vi "TLB Native Dynamic Events ver 0.16a.vi"() -> ()   [LabVIEW 2018]
uses:
  Labview Training Phase 2/Enum Controls/States for Action Engine.ctl
  TLB Type Definitions/State Type Definitions.ctl
  TLB Type Definitions/Intruction Type Definitions.ctl
  TLB Type Definitions/Encoder cluster.ctl
  TLB Type Definitions/PING CLUSTER.ctl
  <vilib>/Studica/Studica Toolkit/NavX/NavX.lvlib
  <vilib>/Studica/Studica Toolkit/Background/DIO Channel.ctl
  Underlying VI's/NavX VI/navX type def.ctl
  <vilib>/myRIO/Instrument Drivers/Utilities/Utilities.lvlib
  <vilib>/Studica/Studica Toolkit/Background/I2C Channel.ctl
  TLB Type Definitions/Vision cluster.ctl
  <vilib>/NI_Real-Time Target Support.lvlib
  TLB Type Definitions/Stepper cluster.ctl
  Experimental VI's/Archived VI's/MOTOR CONTROL NO PID Type Def.ctl
  Underlying VI's/I2C Master VI/I2C MASTER Type Def.ctl
  Underlying VI's/I2C Master VI/I2C_MASTER_WRITE_NEW Type Def.ctl
  <vilib>/userdefined/High Color/IMAQdx.ctl
  Underlying VI's/I2C Master VI/Arduino_Interfacing.ctl
  TLB Type Definitions/Yaw Cluster.ctl
  TLB Type Definitions/Time cluster.ctl
  TLB Type Definitions/Y Stepper cluster.ctl
  Underlying VI's/Modified webcam FGV/Webcam AE.ctl
  Underlying VI's/Elasped Timer/Elapsed timer control.ctl
  Underlying VI's/Motor Control VI with PID/MOTOR CONTROL WITH PID AE DATA MODE TYPE DEF.ctl
  Underlying VI's/Motor Control VI with PID/MOTOR CONTROL WITH PID AE DIRECTION TYPE DEF.ctl
  TLB Type Definitions/IR Sensor Type Def.ctl
  <vilib>/myRIO/Common/Instrument Driver Framework/myRIO v1.0/AI/typedefs/AI Channels Enum.ctl
  <vilib>/myRIO/Common/Instrument Driver Framework/myRIO v1.0/AI/typedefs/AI Channels List.ctl
  <vilib>/Utility/RT CPU Load.ctl
panel:
  out "Left IR Sensor":dbl
  out "Obstacle detected":bool
  out "Speed & distance":T1
  out "Object Center Coordinates":cluster{"x":sgl, "y":sgl}
  out "Object detection cluster":T2
  out "Time up flag":bool
  out "Task selection":u8
  in  "Object recognition mode":enum16{"Ball", "Soap", "Gel", "Pipe", "None"}(ring)
  out "NavX Readings":T3
  out "Arduino Data":T4
  out "CPU loads":T5[](array[typedef]) {"ISR (%)" format="%#.2f"; "Idle (%)" format="%#.2f"; "Background (%)" format="%#.2f"; "Normal (%)" format="%#.2f"; "Above Normal (%)" format="%#.2f"; "High (%)" format="%#.2g"; "Timed Structures (%)" format="%#.2g"; "Time Critical (%)" format="%#.2g"; "Total (%)" format="%#.2g"}
  out "TASK ENABLE":bool
  out "Rising Edge":bool
  in  "Green LED":bool
  out "I2C Error":errorcluster
  out "State Logic":T6=enum."Startup"
  out "elements":T7[](array[typedef])
  in  "STOP TASK":bool
  in  "OK Button":bool
  in  "STOP":bool
  out "error out":errorcluster
  out "Action Queue Items":i32
  out "State Logic Queue Items":i32
  out "Action Queues items":string[](array[string])=["Hardware reset", "Software reset", ""]
  out "Action State":string
  # "System Health Status Update"
  # "VISION"
  # "TLB FRAMEWORK STATUS"
  # "Test Programme written by Calvin Loke    Dated: 28 Aug 2019\nTest Programme revised by Dr Alex See   Dated 30 Aug 2019\n\nRevision date: 20/03/2020\nProgramme version:   TLB Native Dynamic Events ver 0.14a"
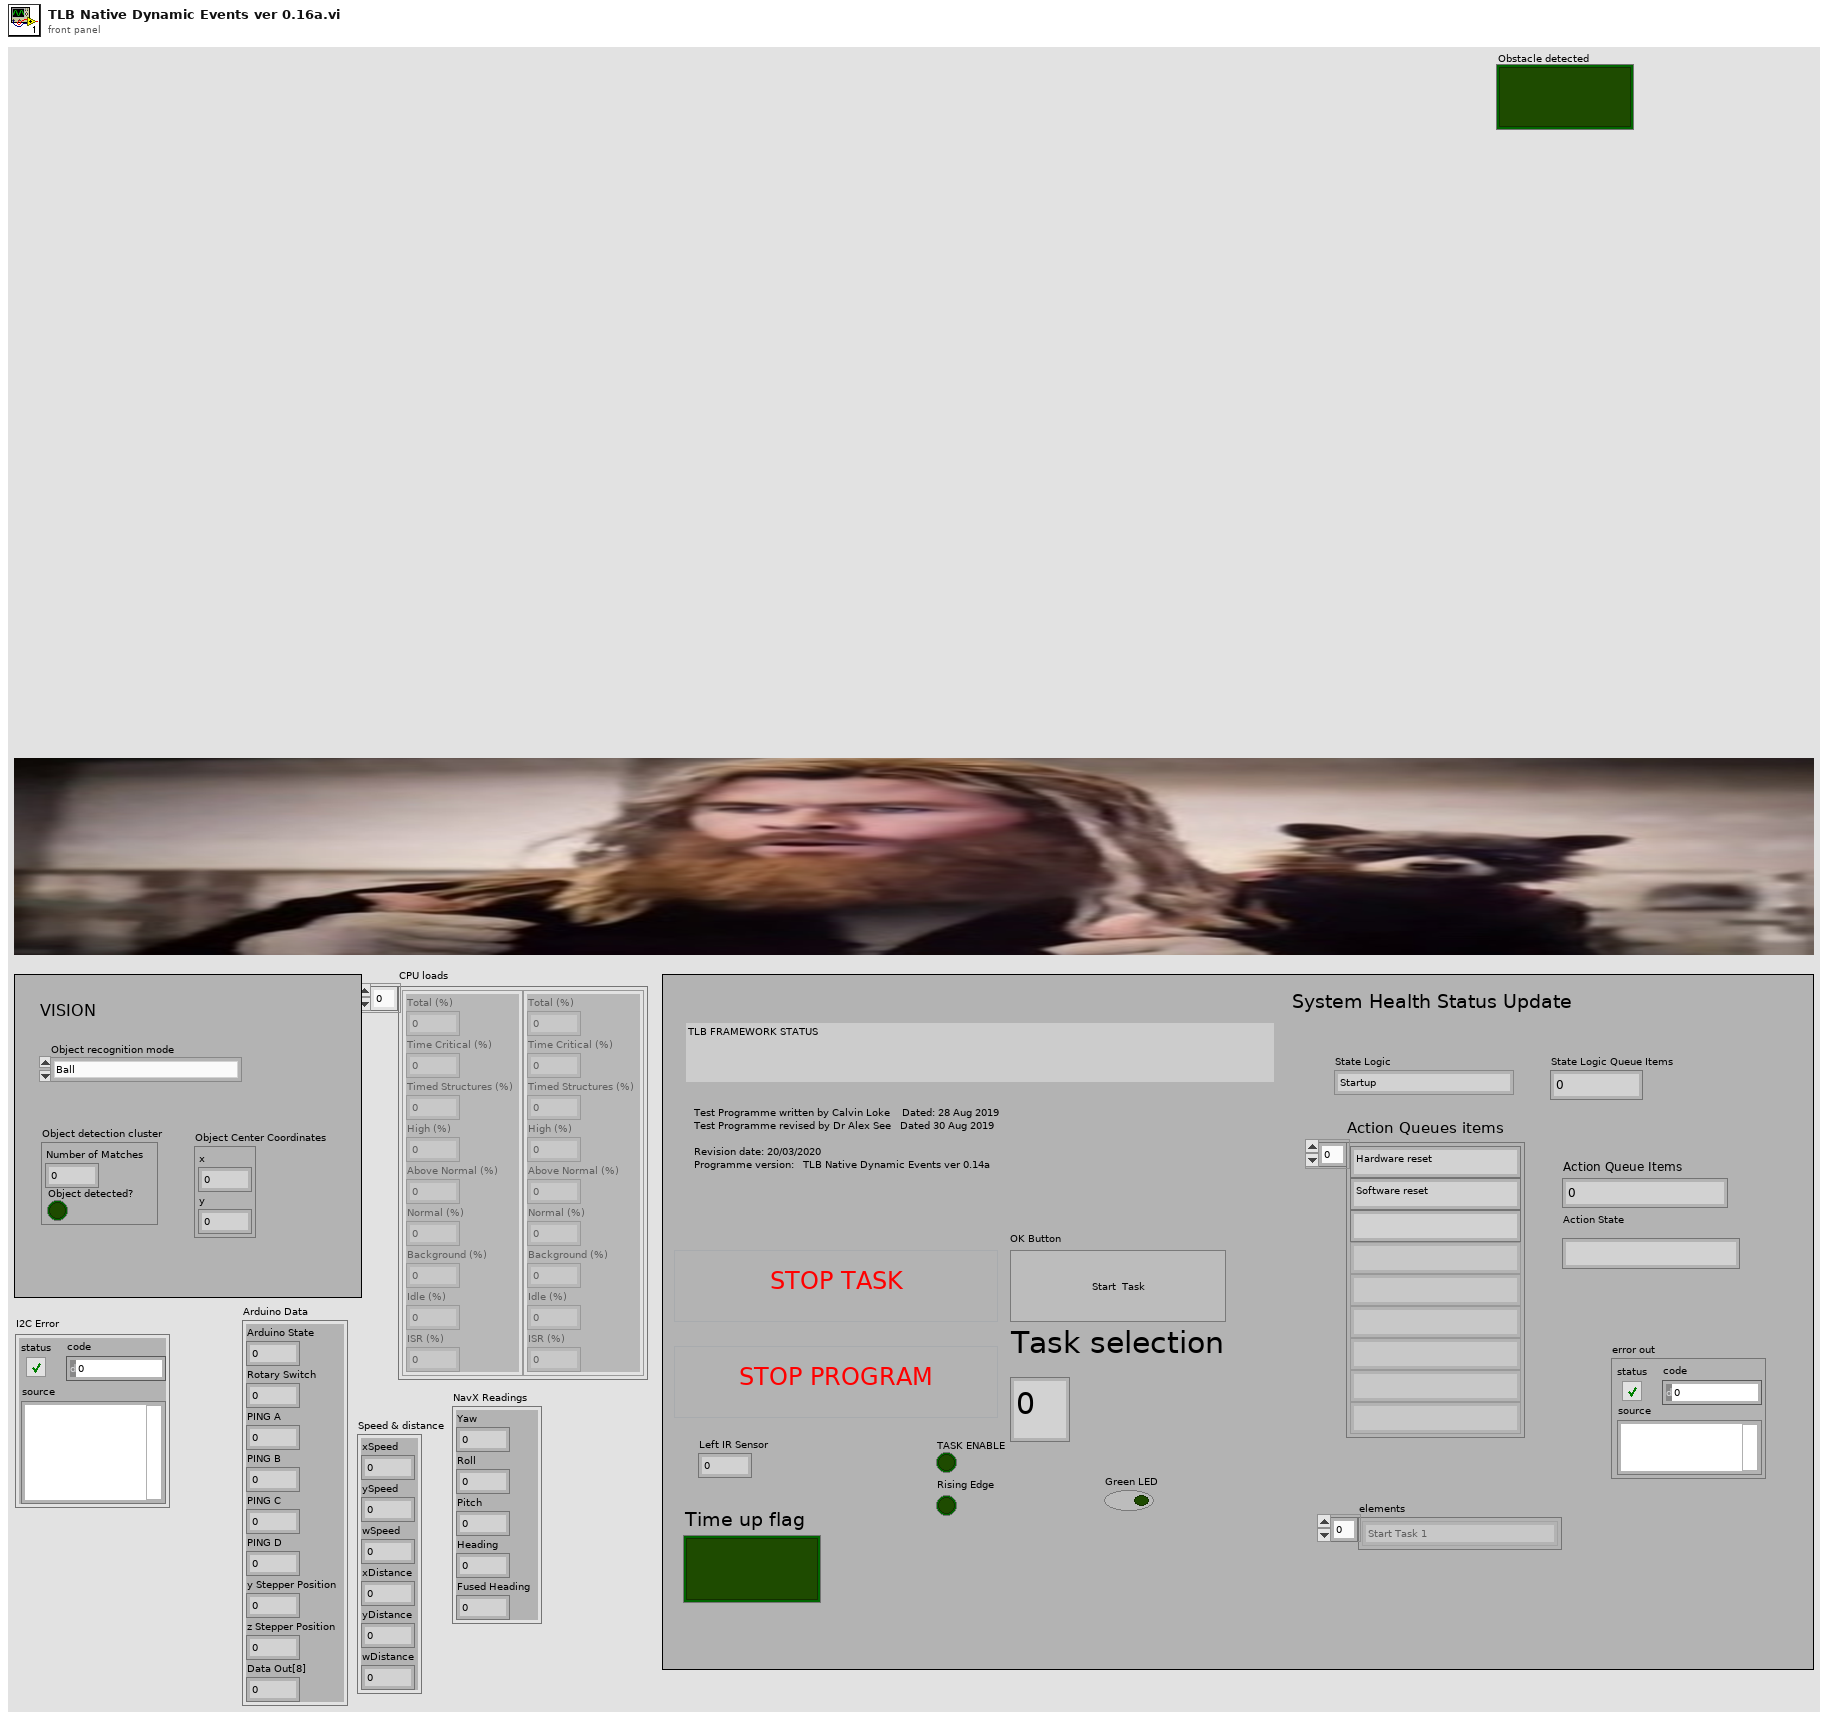
[diagram p1: front panel]
types:
  T1 = cluster{"xSpeed":dbl, "ySpeed":dbl, "wSpeed":dbl, "xDistance":dbl, "yDistance":dbl, "wDistance":dbl}
  T2 = cluster{"Number of Matches":i32, "Object detected?":bool}
  T3 = cluster{"Yaw":dbl, "Roll":dbl, "Pitch":dbl, "Heading":dbl, "Fused Heading":dbl}
  T4 = cluster{"Arduino State":u8, "Rotary Switch":u8, "PING A":u8, "PING B":u8, "PING C":u8, "PING D":u8, "y Stepper Position":u8, "z Stepper Position":u8, "Data Out[8]":u8}
  T5 = typedef "NI_Real-Time Target Support.lvlib/RT CPU Load.ctl" = cluster{"Total (%)":dbl, "Time Critical (%)":dbl, "Timed Structures (%)":dbl, "High (%)":dbl, "Above Normal (%)":dbl, "Normal (%)":dbl, "Background (%)":dbl, "Idle (%)":dbl, "ISR (%)":dbl}
  T6 = typedef "State Type Definitions.ctl" = enum16{"None", "Startup", "Move to Angle", "True Stop", "Idle", "Shutdown", "Task 1A", "Task 1B", "Task 2:Raise Arm", "Task 2:Sensor Mode", "Task 2:Reverse Mode", "Task 3", "Task 4_A", "Task 4_B", "Task 4_C", "Task 4_D", "Task 5A", "Task 5B", "Task 5C", "Task 5D", "Task 5E: POSITION ARM", "Task 5F: ARM GRAB HEIGHT", "Task 5G: CLOSE CLAW", "Task 5H: RAISE ARM", "Task 6_A", "Task 6_B", "Task 7", "Task 8A: RAISE ARM", "Task 8B: MOVE TO BOX", "Task 8C: CAM BURST", "Task 8D: PROCESS IMAGE", "Task 8E: ROBOT ADJUST", "Task 8F: CAM BURST 2", "Task 8G: PROCESS IMAGE 2", "Task 8H: ARM ADJUST", "Task 8I: ARM GRAB HEIGHT", "Task 8J: CLOSE CLAW", "Task 8K: RAISE MY SWORD", "Task 9A: Raise Arm", "Task 9B: Rotate to Angle", "Task 9C: Detect Box", "Task 9D: MOVE FORWARD", "Task 9E: MOVE LEFT", "Task 9F: SCAN IMAGE", "Task 9G: PROCESS COLOUR", "Task 9H: MOVE RIGHT", "Task 9I: SCAN IMAGE", "Task 9J: PROCESS COLOUR", "Task 9K: ROTATE 90 CW", "Task 9L: MOVE FORWARD", "Task 9M: MOVE RIGHT", "Task 9N: SCAN IMAGE", "Task 9O: PROCESS COLOUR", "Task 9P: MOVE RIGHT", "Task 9Q: SCAN IMAGE", "Task 9R: PROCESS COLOUR", "Task A1: Raise Arm", "Task A2: Rotate to Angle", "Task A3: Move Forward", "Task A4: Rotate CW 90"}
  T7 = typedef "Intruction Type Definitions.ctl" = enum16{"None", "Start Task 1", "Start Task 2", "Start Task 3", "Start Task 4", "Start Task 5", "Start Task 6", "Start Task 7", "Start Task 8 - BALL", "Start Task 8 - Gel", "Start Task 8 - Pipe", "Start Task 8 - Soap", "Start Task 9", "Start Task A", "Start Task B", "Exit"}
  T8 = typedef "IR Sensor Type Def.ctl" = cluster{"Left IR Sensor":dbl, "Arm IR Sensor":dbl, "Bottom IR Sensor":dbl}
  T9 = typedef "Y Stepper cluster.ctl" = cluster{"yStepper desired":u8}
  T10 = typedef "Time cluster.ctl" = cluster{"Time up flag":bool, "SET TIME TO CHECK":dbl}
  T11 = typedef "Yaw Cluster.ctl" = cluster{"Yaw":dbl, "Compass":dbl}
  T12 = typedef "Stepper cluster.ctl" = cluster{"y Stepper Position":u8, "z Stepper Position":u8}
  T13 = typedef "DIO Channel.ctl" = enum16{"Not Connected", "A/DIO1", "A/DIO2", "A/DIO3", "A/DIO4", "A/DIO5", "A/DIO6", "A/DIO7", "A/DIO13", "B/DIO1", "B/DIO2", "B/DIO3", "B/DIO4", "B/DIO5", "B/DIO6", "B/DIO7", "B/DIO13", "C/DIO0", "C/DIO1", "C/DIO2", "C/DIO3", "C/DIO4", "C/DIO5", "C/DIO6", "C/DIO7"}
  T14 = typedef "Vision cluster.ctl" = cluster{"Recognized Object":bool, "Object X coordinate":dbl, "Object Y coordinate":dbl}
  T15 = typedef "PING CLUSTER.ctl" = cluster{"PING_A":u8, "PING_B":u8, "PING_C":u8, "PING_D":u8}
  T16 = typedef "Encoder cluster.ctl" = cluster{"xDistance":dbl, "yDistance":dbl, "wDistance":dbl}
  T17 = cluster{"DIO Channel":T13, "FPGA VI Reference Out":refnum<k20>}
  T18 = typedef "navX type def.ctl" = enum16{"Get i2C reference", "Read Values", "Zero Yaw"}
  T19 = typedef "Arduino_Interfacing.ctl" = enum16{"Initialize", "Write to Arduino", "Read From Arduino"}
  T20 = typedef "I2C Channel.ctl" = enum16{"Not Connected", "A", "B"}
  T21 = typedef "States for Action Engine.ctl" = enum16{"Initialize", "Write", "Read"}
  T22 = cluster{"I2C Ref Out":cluster{"I2C Channel":T20, "FPGA VI Reference Out":refnum<k20>}, "Connected":bool, "Slave Address (7-bit)":u8, "Registry":u8[]}
  T23 = typedef "IMAQ Image.ctl" = refnum<image>
  T24 = typedef "State Type Definitions.ctl" = enum16{"None", "Startup", "Move to Angle", "True Stop", "Idle", "Shutdown", "Task 1", "Task 2:Raise Arm", "Task 2:Sensor Mode", "Task 3", "Task 4_A", "Task 4_B", "Task 4_C", "Task 4_D", "Task 5_A", "Task 5 _B", "Task 5_C", "Task 5_D", "Task 5_D_Error", "Task 5D_Error_Right", "Task 5D_Error_Left", "Task 5_E", "Task 5_F", "Task 5F_Error", "Task 5G", "Task 5H", "Task 5I", "Task 6_A", "Task 6_B", "Task 7", "Task 8", "Task 9A: Raise Arm", "Task 9B: Rotate to Angle", "Task 9C: Rotation alignmnet", "Task B"}
  T25 = typedef "MOTOR CONTROL WITH PID AE DIRECTION TYPE DEF.ctl" = enum16{"y-axis movement", "x-axis movement", "rotation", "stop", "reset encoders"}
  T26 = typedef "MOTOR CONTROL WITH PID AE DATA MODE TYPE DEF.ctl" = enum16{"Init AE", "Write to AE", "Read from AE"}
  T27 = typedef "Elapsed timer control.ctl" = enum16{"Start", "Pause", "Initialize"}
  T28 = typedef "I2C_MASTER_WRITE_NEW Type Def.ctl" = enum16{"Ultrasonic sensors", "Stepper origin", "zStepper 13.3k", "zStepper 13k", "zStepper 12k", "zStepper 11k", "zStepper 10k", "zStepper 9k", "zStepper 8k", "zStepper 7k", "zStepper 6k", "zStepper 5k", "zStepper 4k", "zStepper 3k", "zStepper 2k", "zStepper 1k", "zStepper 900", "zStepper 800", "zStepper 700", "zStepper 600", "zStepper 500", "zStepper 400", "zStepper 300", "zStepper 200", "zStepper 100", "zStepper 0", "yStepper control", "Open Claw", "Close Claw", "Soft Reset"}
  T29 = typedef "Webcam AE.ctl" = enum16{"Initialize Camera", "Open Camera", "Continuous Acquisition", "Close Camera", "Retrieve Image", "Dispose Camera Image Buffer"}
  T30 = typedef "IMAQdx.ctl" = refnum<k21>
  T31 = typedef "Webcam AE.ctl" = enum16{"Initialize Camera", "Open Camera", "Continuous Acquisition", "Close Camera", "Retrieve Image", "Dispose Image Buffers"}
  T32 = typedef "MOTOR CONTROL NO PID Type Def.ctl" = enum16{"Init", "Front Back", "Left Right", "Rotate", "Stop", "Latch"}
  T33 = typedef "AI Channels List.ctl" = T34[]
  T34 = typedef "AI Channels Enum.ctl" = enum16{"Not Connected", "AudioIn/Left", "AudioIn/Right", "C/AI0", "C/AI1", "A/AI0", "A/AI1", "A/AI2", "A/AI3", "A/AI4", "A/AI5", "A/AI6", "A/AI7", "B/AI0", "B/AI1", "B/AI2", "B/AI3", "B/AI4", "B/AI5", "B/AI6", "B/AI7", "AI/AI0", "AI/AI1", "AI/AI2", "AI/AI3", "A/AI0 (DIFF)", "A/AI1 (DIFF)", "A/AI2 (DIFF)", "A/AI3 (DIFF)", "B/AI0 (DIFF)", "B/AI1 (DIFF)", "B/AI2 (DIFF)", "B/AI3 (DIFF)"}
  T35 = typedef "I2C MASTER Type Def.ctl" = enum16{"Last State", "Mode 0", "Mode 1", "Mode 2", "Mode 3", "Mode 4", "Mode 5", "Mode 6", "Mode 7", "Mode 8", "Mode 9", "Mode 10"}
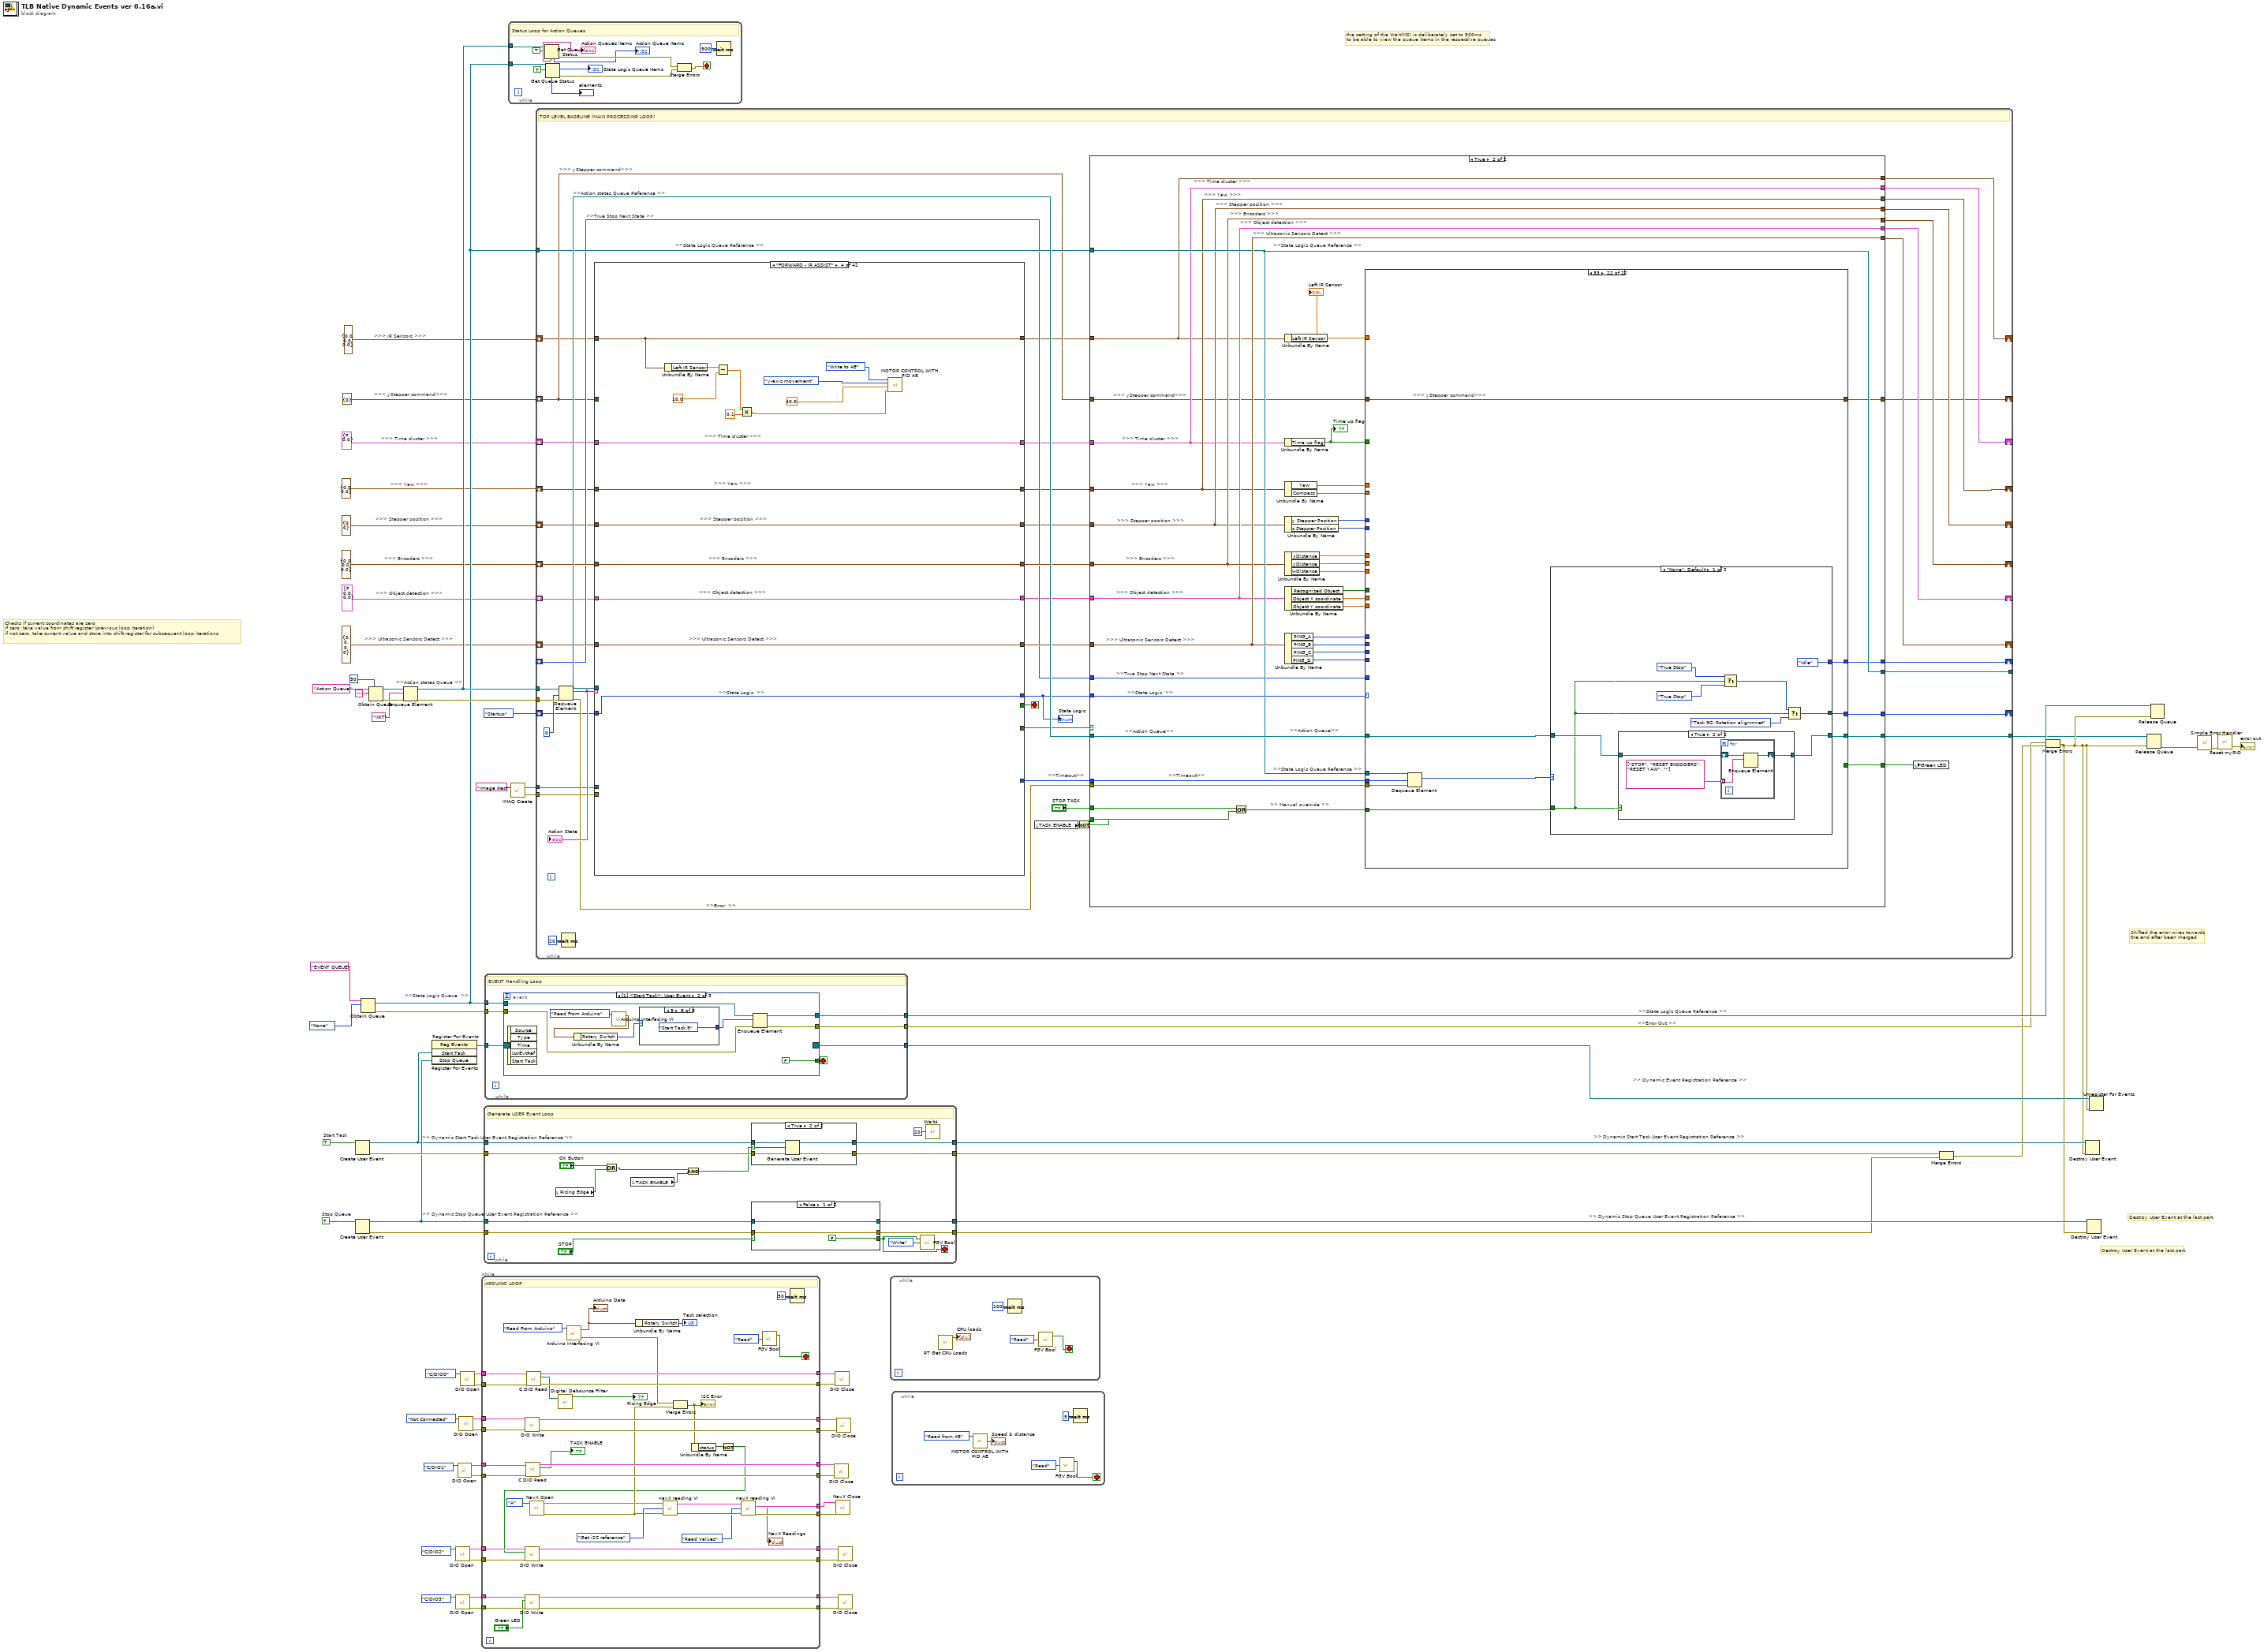
[diagram p0: block diagram]
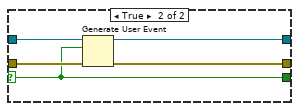
[diagram p2: hidden frame]
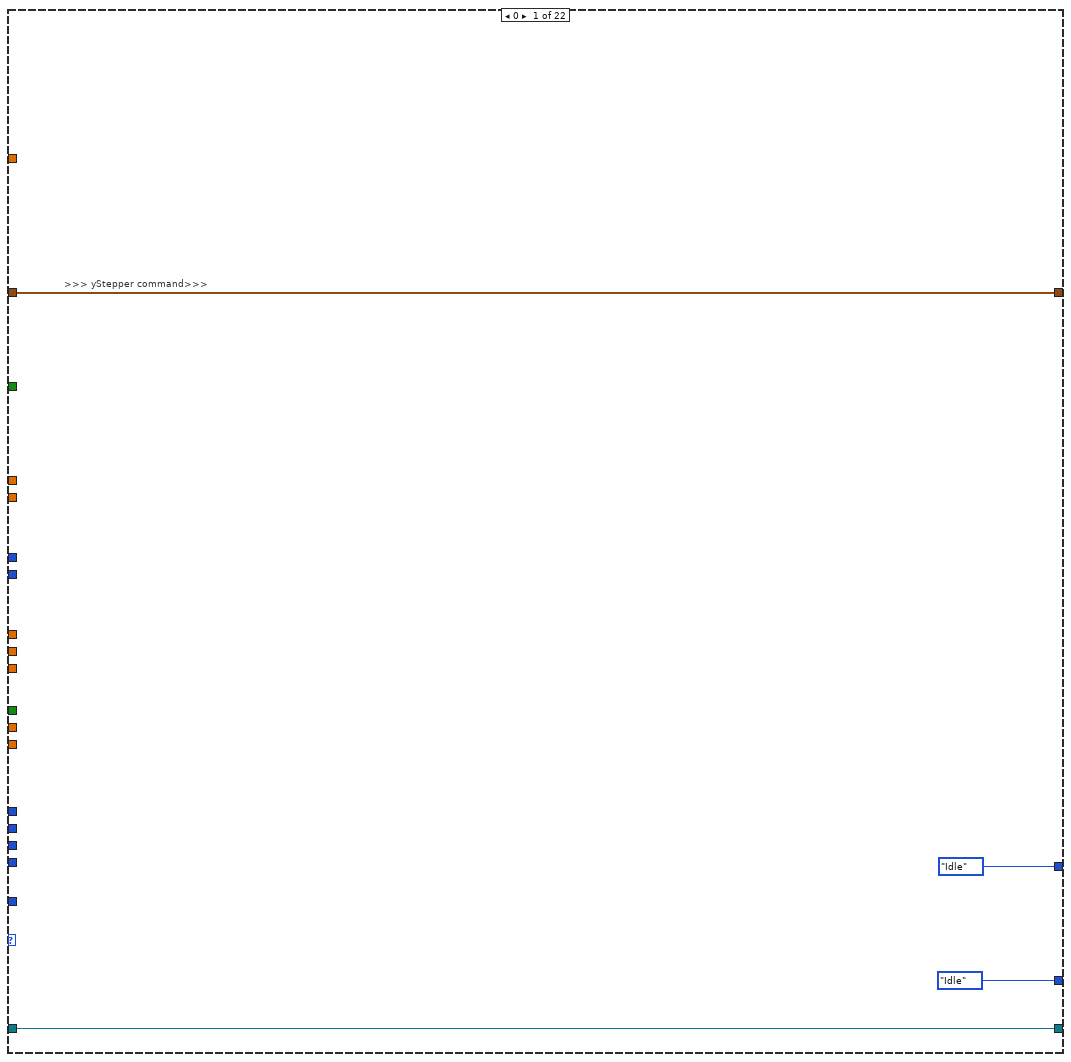
[diagram p5: hidden frame]
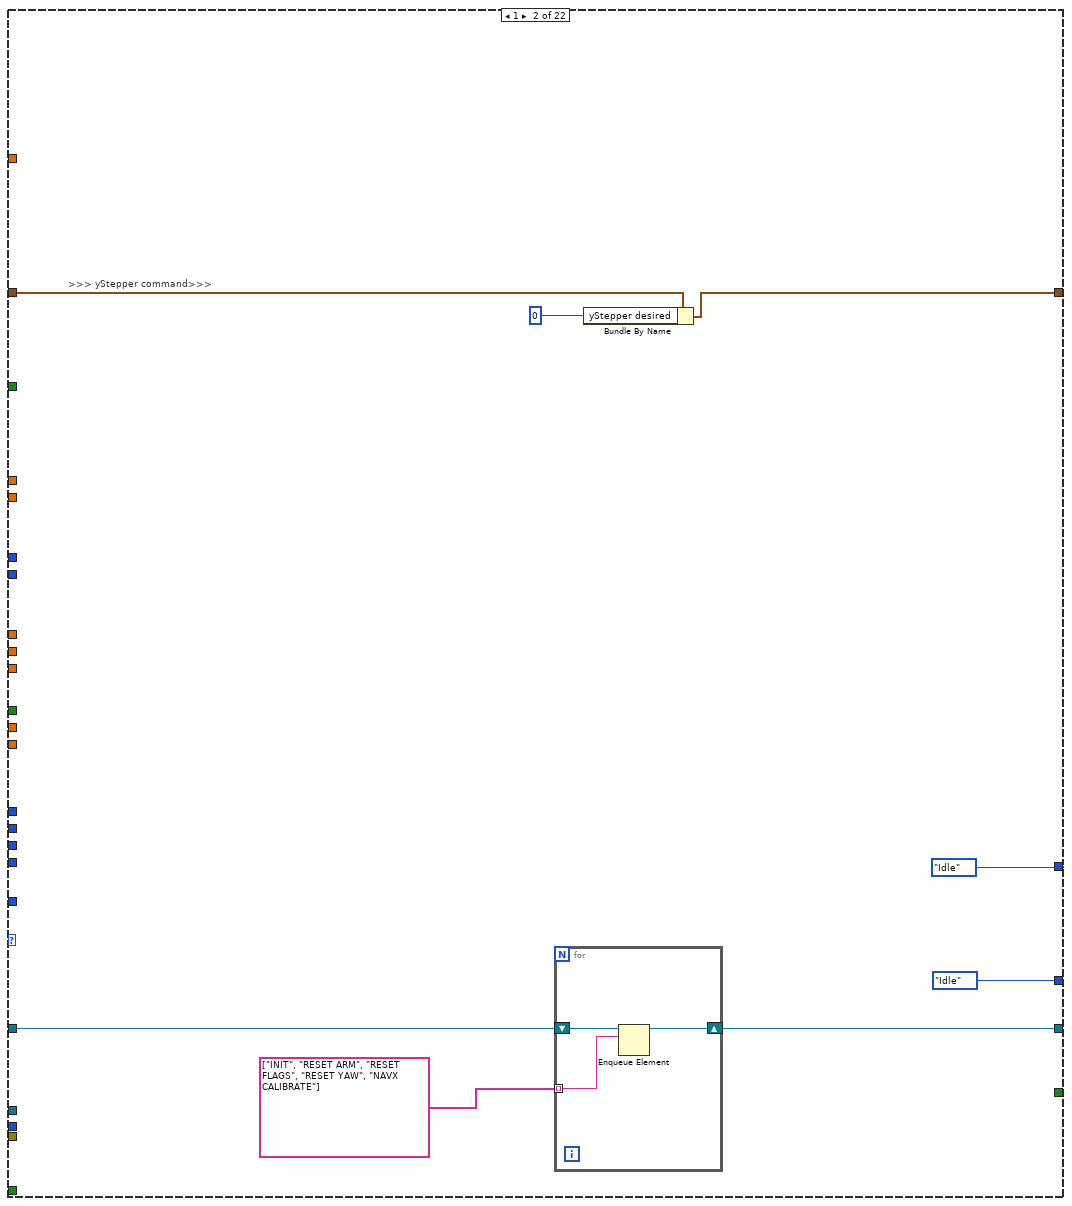
[diagram p6: hidden frame]
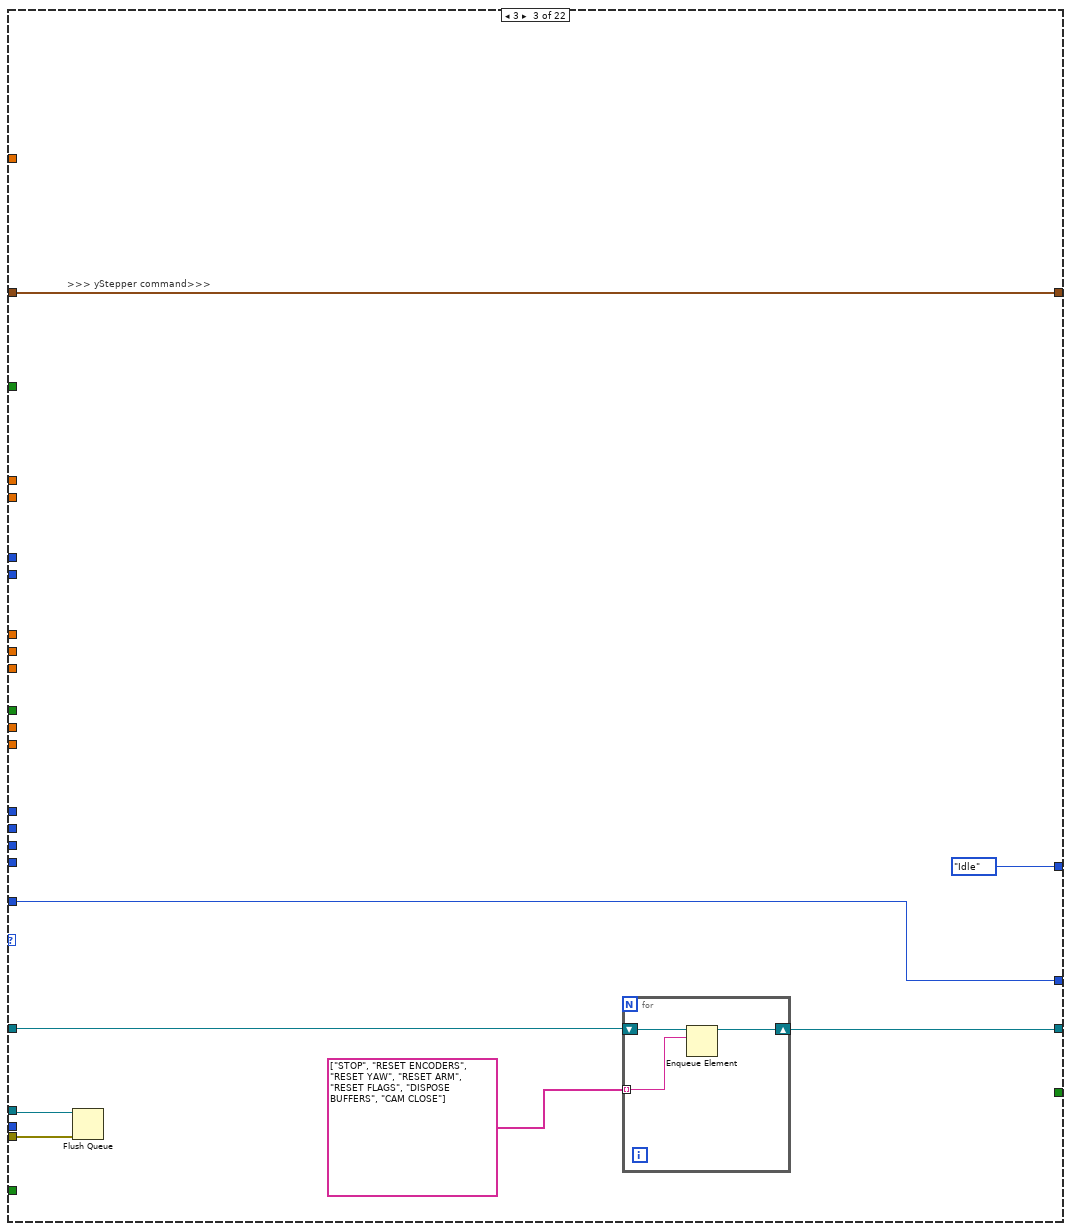
[diagram p7: hidden frame]
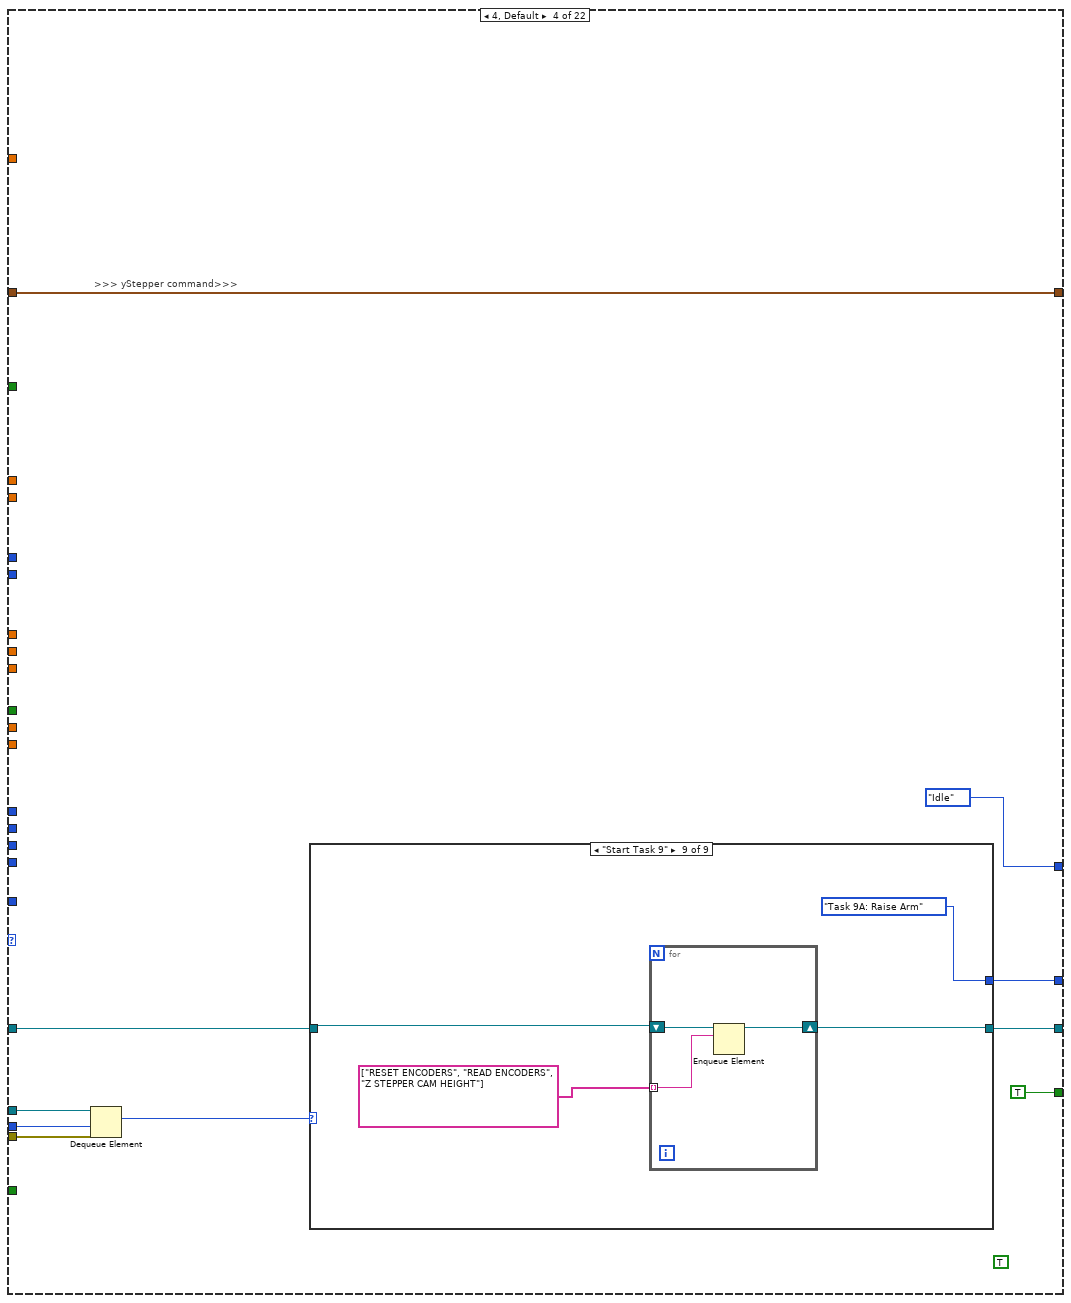
[diagram p8: hidden frame]
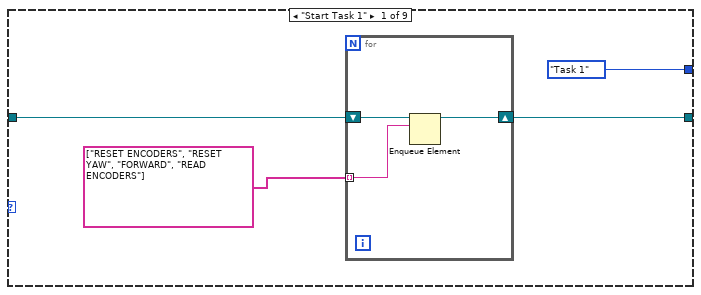
[diagram p9: hidden frame]
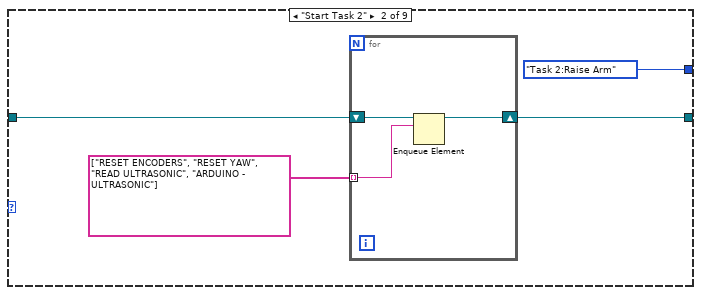
[diagram p10: hidden frame]
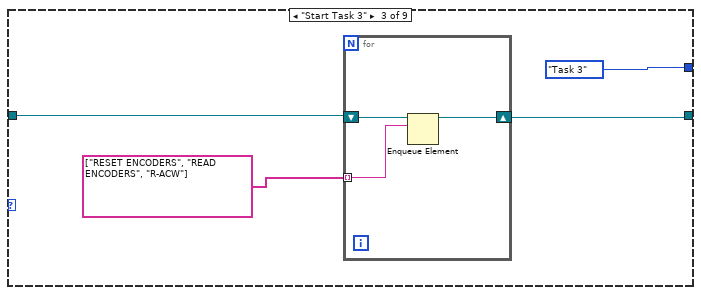
[diagram p11: hidden frame]
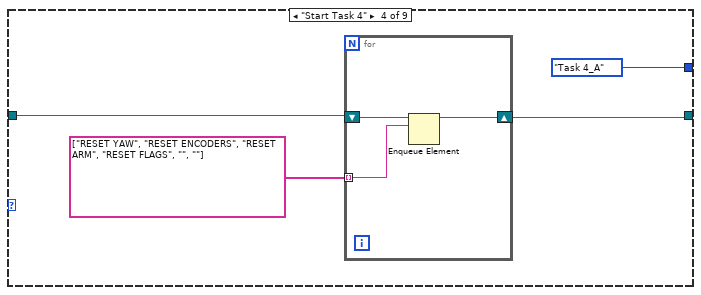
[diagram p12: hidden frame]
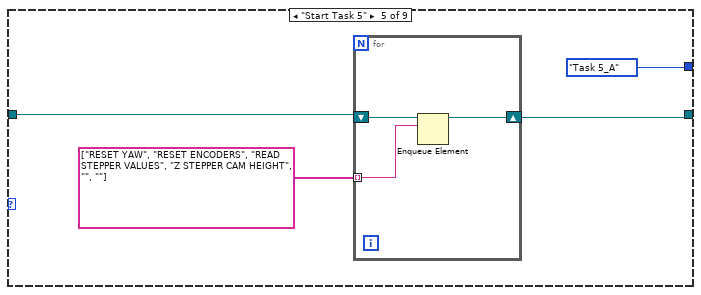
[diagram p13: hidden frame]
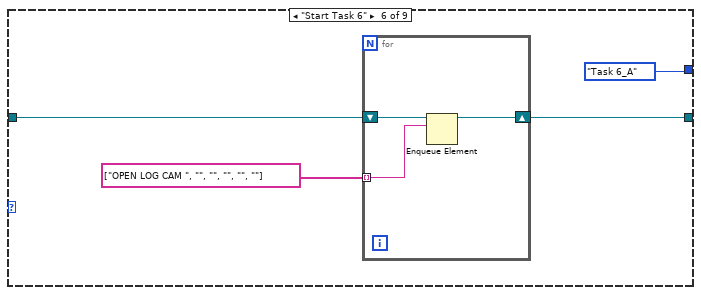
[diagram p14: hidden frame]
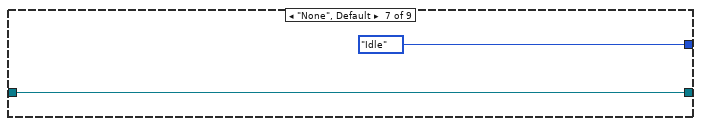
[diagram p15: hidden frame]
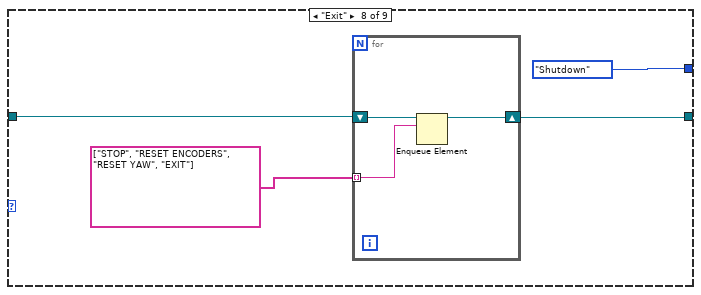
[diagram p16: hidden frame]
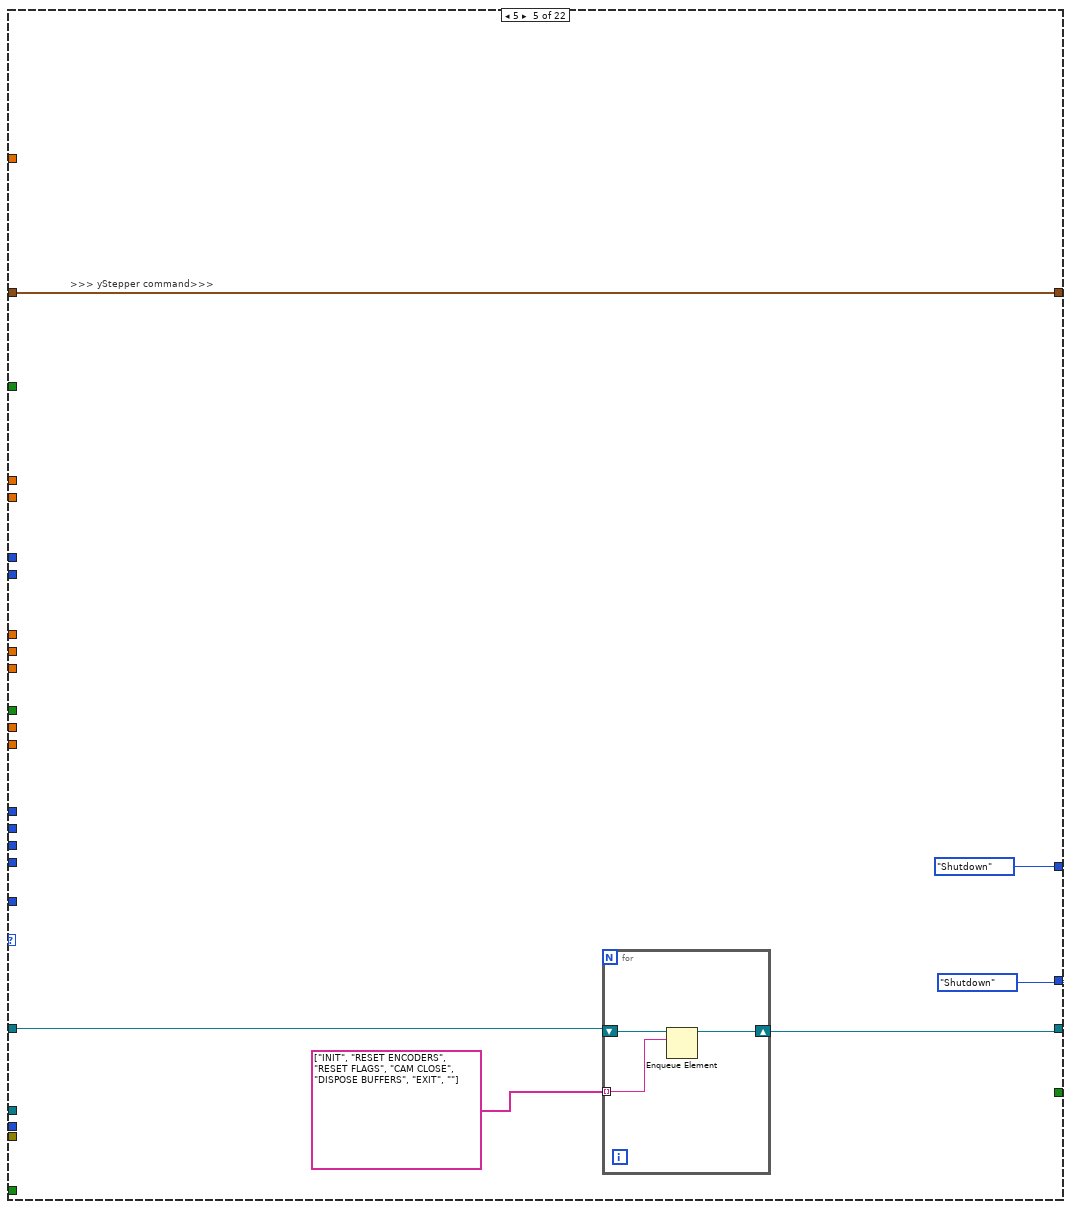
[diagram p17: hidden frame]
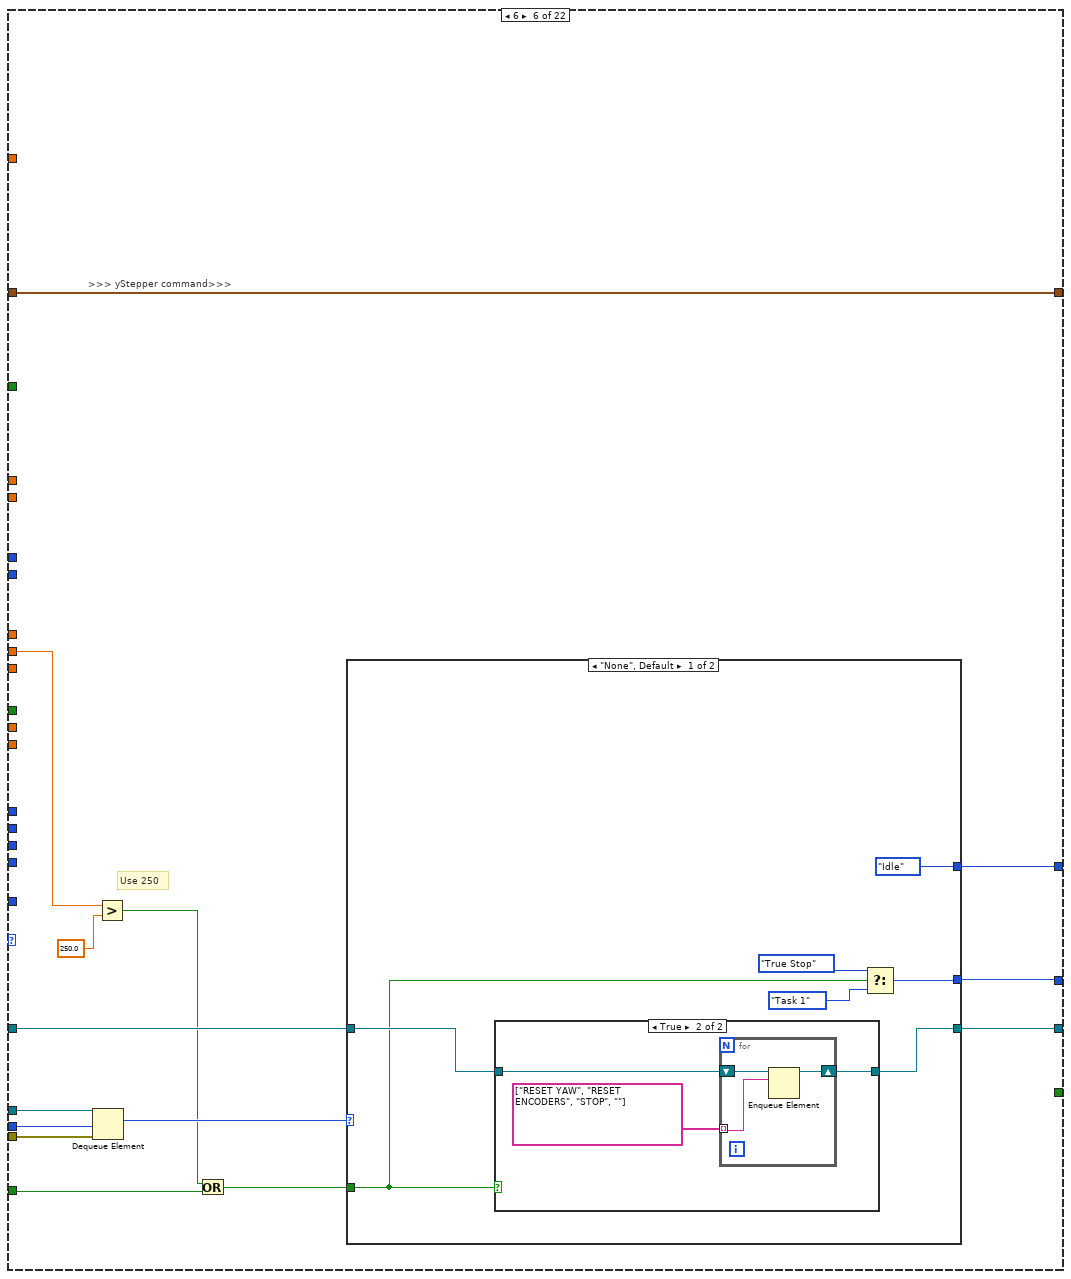
[diagram p18: hidden frame]
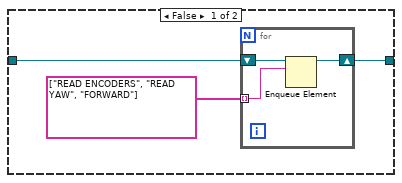
[diagram p19: hidden frame]
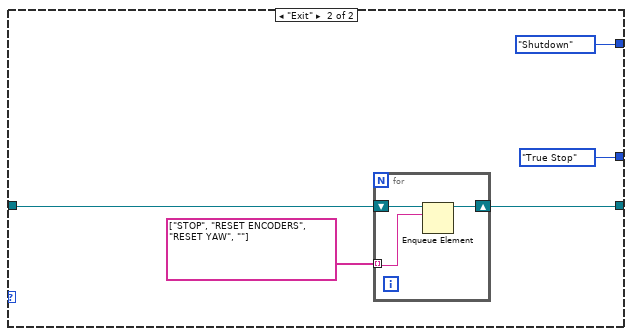
[diagram p20: hidden frame]
diagram:
  w71 = TRUE  # Stop Queue
  w70 = TRUE  # Start Task
  # ">>> IR Sensors >>>"
  # "Checks if current coordinates are zero\nif zero, take value from shift register (previous loop iteration)\nif not zero, take current value and store into shift register for subsequent loop iterations"
  # ">>> yStepper command>>>"
  # ">>> Time cluster >>>"
  # ">>> Yaw >>>"
  # ">>> Stepper position >>>"
  # ">>> Encoders >>>"
  # ">>> Object detection >>>"
  # ">>> Ultrasonic Sensors Detect >>>"
  # "the setting of the Wait(MS) is deliberately set to 500ms\nto be able to view the queue items in the respective queues"
  # ">>Error Out >>"
  # ">> Dynamic Stop Queue User Event Registration Reference >>"
  # ">> Dynamic Start Task User Event Registration Reference >>"
  # ">> Dynamic Stop Queue User Event Registration Reference >>"
  # ">> Dynamic Start Task User Event Registration Reference >>"
  # ">> Dynamic Event Registration Reference >>"
  # ">>Action states Queue >>"
  # ">>State Logic Queue  >>"
  # ">>State Logic Queue Reference >>"
  # "Destroy User Event at the last part"
  # "Destroy User Event at the last part"
  # "Shifted the error wires towards\nthe end after been merged"
  n1 = Create User Event(user event datatype=w70) -> (user event=w62:refnum<user-event>, error out=w67:errorcluster)  [unwired: 1 in]
  n2 = Create User Event(user event datatype=w71) -> (user event=w63:refnum<user-event>, error out=w66:errorcluster)  [unwired: 1 in]
  n3 = Obtain Queue(name (unnamed)="EVENT QUEUE", element data type=Intruction_Type_Definitions."None" ("Enum")) -> (queue out=w48:refnum<queue>, error out=w54:errorcluster)  [unwired: 3 in, 1 out]
  n4 = Obtain Queue(max queue size (-1, unlimited)=50, name (unnamed)="Action Queue", element data type="") -> (queue out=w57:refnum<queue>, error out=w53:errorcluster)  [unwired: 2 in, 1 out]
  n5 = Enqueue Element(queue=w57, element="INIT", error in (no error)=w53) -> (queue out=w49:refnum<queue>, error out=w52:errorcluster)  [unwired: 1 in, 1 out]
  n6 = register-events "Register For Events"(w62, w63) -> (reference out=w61:refnum<event-registration>)  [unwired: 2 in, 1 out]
  n7 = call <vilib>:"DIO Open.vi"("DIO Channel"=DIO_Channel."C/DIO2") -> ("error out"=w15:errorcluster, "DIO Info Out"=w16:T17)  [unwired: 9 in]
  n8 = call <vilib>:"DIO Open.vi"("DIO Channel"=DIO_Channel."C/DIO3") -> ("error out"=w10:errorcluster, "DIO Info Out"=w11:T17)  [unwired: 9 in]
  n9 = call <vilib>:"DIO Open.vi"("DIO Channel"=DIO_Channel."C/DIO1") -> ("error out"=w26:errorcluster, "DIO Info Out"=w27:T17)  [unwired: 9 in]
  n10 = call <vilib>:"DIO Open.vi"("DIO Channel"=DIO_Channel."Not Connected") -> ("error out"=w31:errorcluster, "DIO Info Out"=w33:T17)  [unwired: 9 in]
  n11 = call <vilib>:"DIO Open.vi"("DIO Channel"=DIO_Channel."C/DIO0") -> ("error out"=w36:errorcluster, "DIO Info Out"=w39:T17)  [unwired: 9 in]
  n12 = while {
    tunnel: w39 -> [w112]
    tunnel: [w111] -> w37
    tunnel: w36 -> [w110]
    tunnel: [w109] -> w35
    tunnel: w33 -> [w106]
    tunnel: [w105] -> w32
    tunnel: w31 -> [w104]
    tunnel: [w103] -> w30
    tunnel: [w102] -> w28
    tunnel: w27 -> [w101]
    tunnel: w26 -> [w100]
    tunnel: [w99] -> w25
    tunnel: w16 -> [w93]
    tunnel: w15 -> [w92]
    tunnel: [w91] -> w14
    tunnel: [w90] -> w13
    tunnel: w11 -> [w89]
    tunnel: w10 -> [w88]
    tunnel: [w87] -> w9
    tunnel: [w86] -> w8
    tunnel: [w80] -> w5
    tunnel: [w79] -> w6
    stop <- w114 stop-if-true
    # "ARDUINO LOOP"
    n13 = call <vilib>:"DIO Write.vi"("error in (no error)"=w88, "Input"="Green LED", "DIO Info In"=w89) -> ("error out"=w86:errorcluster, "DIO Info Out"=w87:T17)  [unwired: 7 in]
    n14 = call <vilib>:"DIO Write.vi"("error in (no error)"=w104, "DIO Info In"=w106) -> ("error out"=w103:errorcluster, "DIO Info Out"=w105:T17)  [unwired: 8 in]
    n15 = call <vilib>:"C DIO Read.vi"("error in (no error)"=w100, "DIO Info In in"=w101) -> ("error out"=w99:errorcluster, "IN"=→"TASK ENABLE":bool, "DIO Info In out"=w102:T17)  [unwired: 7 in]
    n16 = call <vilib>:"C DIO Read.vi"("error in (no error)"=w110, "DIO Info In in"=w112) -> ("error out"=w109:errorcluster, "IN"=w108:bool, "DIO Info In out"=w111:T17)  [unwired: 7 in]
    n17 = call <vilib>:"NavX Open.vi"("I2C Channel"=I2C_Channel."A") -> ("error out"=w95:errorcluster, "NavX Info"=w97:T22)  [unwired: 9 in]
    n18 = call "Digital Debounce Filter.vi"("Boolean input"=w108) -> ("Rising Edge"=→"Rising Edge":bool)  [unwired: 1 in, 2 out]
    n19 = call "Arduino Interfacing VI.vi"("AE Mode"=Arduino_Interfacing."Read From Arduino") -> ("error out"=w83:errorcluster, "Arduino Data"=w76:T4)  [unwired: 3 in]
    "Arduino Data" <- w76
    n20 = Unbundle By Name(w76) -> ("Rotary Switch"=→"Task selection":u8)
    n21 = call "navX reading VI.vi"("NavX Info In"=w97, "Mode"=navX_type_def."Get i2C reference", "error in (no error)"=w95) -> ("NavX Info Out"=w82:T22, "Error Out"=w81:errorcluster)  [unwired: 2 out]
    n22 = Merge Errors(w83, w95) -> (w74:errorcluster)
    "I2C Error" <- w74
    n23 = Unbundle By Name(w74) -> ("status"=w73:bool)
    n24 = Not(x=w73) -> (.not. x?=w72:bool)
    n25 = call <vilib>:"DIO Write.vi"("error in (no error)"=w92, "Input"=w72, "DIO Info In"=w93) -> ("error out"=w90:errorcluster, "DIO Info Out"=w91:T17)  [unwired: 7 in]
    n26 = call "navX reading VI.vi"("NavX Info In"=w82, "Mode"=navX_type_def."Read Values", "error in (no error)"=w81) -> ("NavX Info Out"=w80:T22, "NavX Readings"=→"NavX Readings":T3, "Error Out"=w79:errorcluster)  [unwired: 1 out]
    n27 = call "FGV Bool.vi"("Init/Read/Write State"=States_for_Action_Engine."Read") -> ("Output node"=w114:bool)  [unwired: 2 in, 1 out]
    n28 = Wait (ms)(milliseconds to wait=u32 50) -> ()  [unwired: 1 out]
  }
  n29 = while {
    tunnel: w62 -> [w132]
    tunnel: w63 -> [w131]
    tunnel: [w130] -> w69
    tunnel: [w129] -> w68
    tunnel: w67 -> [w128]
    tunnel: [w127] -> w65
    tunnel: w66 -> [w126]
    tunnel: [w125] -> w64
    stop <- w123 stop-if-true
    # "Generate USER Event Loop"
    n30 = local read "Rising Edge"() -> (w119:bool)
    n31 = Or(x="OK Button", y=w119) -> (x .or. y?=w118:bool)
    n32 = local read "TASK ENABLE"() -> (w117:bool)
    n33 = And(x=w118, y=w117) -> (x .and. y?=w116:bool)
    n34 = case shown="True" w116 {
      selector: w116 -> [_ w143]
      tunnel: w132 -> [w142 w147]
      tunnel: [w142 w146] -> w129
      tunnel: w128 -> [w141 w145]
      tunnel: [w141 w144] -> w127
      frame False {
      }
      frame True {
        n35 = Generate User Event(user event=w147, event data cluster=w143, error in=w145) -> (user event out=w146:refnum<user-event>, error out=w144:errorcluster)  [unwired: 1 in]
      }
    }
    n36 = case shown="False" "STOP" {
      selector: "STOP" -> [_ w136]
      tunnel: w131 -> [w135 w140]
      tunnel: [w135 w139] -> w130
      tunnel: w126 -> [w134 w138]
      tunnel: [w134 w137] -> w125
      tunnel: [FALSE w136] -> w123
      frame False {
      }
      frame True {
        n37 = Generate User Event(user event=w140, event data cluster=w136, error in=w138) -> (user event out=w139:refnum<user-event>, error out=w137:errorcluster)  [unwired: 1 in]
      }
    }
    n38 = call "FGV Bool.vi"("Init/Read/Write State"=States_for_Action_Engine."Write", "Input Node"=w123) -> ()  [unwired: 1 in, 2 out]
    n39 = call "Wait4"("Count(uSec)"=u32 20) -> ()  [unwired: 1 out]
  }
  n40 = while {
    tunnel: w61 -> [w154]
    tunnel: [w153] -> w60
    tunnel: w48 -> [w151]
    tunnel: [w150] -> w59
    tunnel: w54 -> [w149]
    tunnel: [w148] -> w51
    stop <- w152 stop-if-true
    # "EVENT Handling Loop"
    n41 = event shown="[1] <Start Task>: User Event" {
      selector: w154 -> [_ _ _]
      dyn-events: [_ _ _] -> w153
      timeout: _ -> [_ _ _]
      tunnel: [FALSE FALSE w183] -> w152
      tunnel: w151 -> [w159 w168 w181]
      tunnel: [w158 w167 w182] -> w150
      tunnel: w149 -> [w157 w166 w180]
      tunnel: [w156 w165 w179] -> w148
      event Timeout {
        n42 = event-data() -> ()  [unwired: 1 in, 3 out]
        n43 = Enqueue Element(queue=w159, element=Intruction_Type_Definitions."None" ("Enum"), error in (no error)=w157) -> (queue out=w158:refnum<queue>, error out=w156:errorcluster)  [unwired: 1 in, 1 out]
      }
      event User Event {
        n44 = event-data() -> ()  [unwired: 1 in, 5 out]
        n45 = call "Arduino Interfacing VI.vi"("AE Mode"=Arduino_Interfacing."Read From Arduino") -> ("Arduino Data"=w162:T4)  [unwired: 3 in, 1 out]
        n46 = Unbundle By Name(w162) -> ("Rotary Switch"=w161:u8)
        n47 = case shown="9" w161 {
          tunnel: [Intruction_Type_Definitions."None" ("Enum") Intruction_Type_Definitions."Start Task 1" ("Enum") Intruction_Type_Definitions."Start Task 2" ("Enum") Intruction_Type_Definitions."Start Task 3" ("Enum") Intruction_Type_Definitions."Start Task 4" ("Enum") Intruction_Type_Definitions."Start Task 5" ("Enum") Intruction_Type_Definitions."Start Task 6" ("Enum") Intruction_Type_Definitions."Start Task 9" ("Enum")] -> w164
          frame 0, Default {
          }
          frame 1 {
          }
          frame 2 {
          }
          frame 3 {
          }
          frame 4 {
          }
          frame 5 {
          }
          frame 6 {
          }
          frame 9 {
          }
        }
        n48 = Enqueue Element(queue=w168, element=w164, error in (no error)=w166) -> (queue out=w167:refnum<queue>, error out=w165:errorcluster)  [unwired: 1 in, 1 out]
      }
      event User Event {
        n49 = event-data() -> ("Stop Queue"=w183:bool)  [unwired: 1 in, 4 out]
        n50 = Enqueue Element At Opposite End(queue=w181, element=Intruction_Type_Definitions."Exit" ("Enum"), error in (no error)=w180) -> (queue out=w182:refnum<queue>, error out=w179:errorcluster)  [unwired: 1 in, 1 out]
      }
    }
  }
  n51 = while {
    tunnel: w49 -> [w193]
    tunnel: w48 -> [w190]
    stop <- w187 stop-if-true
    # "Status Loop for Action Queues"
    n52 = Get Queue Status(queue=w193, return elements? (F)=TRUE) -> (error out=w189:errorcluster, # elements in queue=→"Action Queue Items":i32, elements=→"Action Queues items":string[])  [unwired: 1 in, 5 out]
    n53 = Get Queue Status(queue=w190, return elements? (F)=TRUE) -> (# pending remove=→"State Logic Queue Items":i32, error out=w188:errorcluster, elements=→"elements":T7[])  [unwired: 1 in, 5 out]
    n54 = Merge Errors(w189, w188) -> (w187:errorcluster)
    n55 = Wait (ms)(milliseconds to wait=u32 500) -> ()  [unwired: 1 out]
  }
  n56 = call "IMAQ Create"("Image Name"="Image dest") -> ("New Image"=w20:T23, "error out"=w19:errorcluster)  [unwired: 4 in]
  n57 = while {
    tunnel: w48 -> [w230]
    tunnel: w49 -> [w242]
    tunnel: w52 -> [w240]
    tunnel: [w239] -> _
    tunnel: [w238] -> w42
    shift-right: [w231] -> _
    shift-left: T15 {"PING_A"=0, "PING_B"=0, "PING_C"=0, "PING_D"=0} -> [w233]
    shift-right: [w224] -> _
    shift-left: State_Type_Definitions."Startup" ("Enum") -> [w227]
    shift-right: [w220] -> _
    shift-left: T16 {"xDistance"=0.0, "yDistance"=0.0, "wDistance"=0.0} -> [w222]
    shift-right: [w217] -> _
    shift-left: _ -> [w216]
    tunnel: w20 -> [w215]
    tunnel: w19 -> [w214]
    shift-right: [w211] -> _
    shift-left: T14 {"Recognized Object"=FALSE, "Object X coordinate"=0.0, "Object Y coordinate"=0.0} -> [w213]
    shift-right: [w208] -> _
    shift-left: T12 {"y Stepper Position"=0, "z Stepper Position"=0} -> [w210]
    shift-right: [w205] -> _
    shift-left: T11 {"Yaw"=0.0, "Compass"=0.0} -> [w207]
    shift-right: [w202] -> _
    shift-left: T10 {"Time up flag"=FALSE, "SET TIME TO CHECK"=0.0} -> [w204]
    shift-right: [w200] -> _
    shift-left: T9 {"yStepper desired"=0} -> [w201]
    shift-right: [w196] -> _
    shift-left: T8 {"Left IR Sensor"=0.0, "Arm IR Sensor"=0.0, "Bottom IR Sensor"=0.0} -> [w198]
    stop <- w229 stop-if-true
    # ">>> yStepper command>>>"
    # ">>True Stop Next State >>"
    # ">>Error  >>"
    # ">>Timeout>>"
    # ">>Action states Queue Reference >>"
    # ">>State Logic Queue Reference >>"
    # "TOP LEVEL BASELINE (MAIN PROCESSING LOOP)"
    n58 = Dequeue Element(queue=w242, timeout in ms (-1)=0, error in (no error)=w240) -> (queue out=w234:refnum<queue>, element=w241:string, error out=w235:errorcluster)  [unwired: 1 out]
    "Action State" <- w241
    n59 = Wait (ms)(milliseconds to wait=u32 20) -> ()  [unwired: 1 out]
    n60 = case shown="\"FORWARD - IR ASSIST\"" w241 {
      tunnel: [_ _ _ _ _ _ _ _ _ _ _ _ _ _ _ _ _ _ 0 w1375 _ _ _ _ _ _ _ _ _ _ _ _ _ _ _ _ _ _ _ _ _ _] -> w237
      tunnel: w234 -> [_ _ _ _ _ _ _ _ _ _ _ _ _ _ _ _ _ _ _ _ _ _ _ _ _ _ _ _ _ _ _ _ _ _ _ _ _ _ _ _ _ _]
      tunnel: w233 -> [w1146 w1155 w1167 w1178 w1195 w1206 w1217 w1229 w1241 w1252 w1259 w1274 w1288 w1300 w1308 w1320 w1345 w1355 w1366 w1376 w1385 w1395 w1425 w1436 w1444 w1453 w1466 w1479 w1489 w1498 w1515 w1524 w1535 w1545 w1555 w1565 w1572 w1584 w1600 w1606 w1618 w1629]
      tunnel: [w1146 w1155 w1167 w1178 w1195 w1206 w1217 w1229 w1241 w1252 w1259 w1274 w1289 w1300 w1308 w1320 w1346 w1355 w1366 w1376 w1385 w1395 w1424 w1436 w1444 w1453 w1466 w1479 w1489 w1498 w1515 w1524 w1535 w1545 w1555 w1565 w1572 w1584 w1600 w1606 w1618 w1629] -> w232
      tunnel: [TRUE TRUE _ _ _ _ _ _ _ _ _ _ _ _ _ _ _ _ _ _ _ _ _ _ _ _ _ _ _ _ _ _ _ _ _ _ _ _ _ _ _ _] -> w229
      tunnel: w227 -> [w1144 w1153 w1166 w1177 w1194 w1205 w1216 w1228 w1240 w1251 w1258 w1273 w1287 w1299 w1306 w1319 w1344 w1354 w1363 w1373 w1384 w1394 w1423 w1435 w1443 w1452 w1465 w1478 w1488 w1497 w1514 w1523 w1534 w1544 w1554 w1564 w1571 w1583 w1599 w1605 w1617 w1628]
      tunnel: [_ _ _ _ _ _ _ _ _ _ _ _ _ _ _ _ _ _ _ TRUE _ _ _ _ _ _ _ _ _ _ _ _ _ _ _ _ _ _ _ _ _ _] -> w226
      tunnel: [w1144 w1153 w1166 w1177 w1194 w1205 w1216 w1228 w1240 w1251 w1258 w1273 w1287 w1299 w1306 w1319 w1344 w1354 w1363 w1373 w1384 w1394 w1423 w1435 w1443 w1452 w1465 w1478 w1488 w1497 w1514 w1523 w1534 w1544 w1554 w1564 w1571 w1583 w1599 w1605 w1617 w1628] -> w225
      tunnel: w222 -> [w1143 w1152 w1165 w1180 w1193 w1204 w1215 w1227 w1239 w1250 w1260 w1272 w1286 w1301 w1310 w1321 w1343 w1356 w1362 w1372 w1386 w1396 w1413 w1434 w1446 w1454 w1467 w1480 w1490 w1499 w1516 w1526 w1537 w1547 w1557 w1567 w1574 w1586 w1602 w1608 w1620 w1631]
      tunnel: [w1143 w1152 w1165 w1180 w1193 w1204 w1215 w1227 w1239 w1250 w1260 w1271 w1286 w1301 w1310 w1321 w1342 w1356 w1362 w1372 w1386 w1396 w1412 w1434 w1446 w1454 w1467 w1480 w1490 w1499 w1516 w1526 w1537 w1547 w1557 w1567 w1574 w1586 w1602 w1608 w1620 w1631] -> w221
      tunnel: w215 -> [w1138 _ _ _ _ _ _ _ _ _ _ _ _ _ _ _ _ _ _ _ _ _ _ _ _ _ _ _ _ _ w1510 _ _ _ _ _ _ _ _ _ _ _]
      tunnel: w214 -> [_ _ _ _ _ _ _ _ _ _ _ _ _ _ _ _ _ _ _ _ _ _ _ _ _ _ _ _ w1482 _ w1512 w1522 _ _ _ _ _ _ _ _ _ _]
      tunnel: w213 -> [w1142 w1151 w1164 w1179 w1192 w1203 w1214 w1226 w1238 w1248 w1257 w1270 w1285 w1294 w1309 w1318 w1334 w1353 w1361 w1371 w1383 w1393 w1418 w1432 w1445 w1451 w1464 w1477 w1484 w1496 w1507 w1525 w1536 w1546 w1556 w1566 w1573 w1585 w1601 w1607 w1619 w1630]
      tunnel: [w1142 w1151 w1164 w1179 w1192 w1203 w1214 w1226 w1238 w1248 w1257 w1270 w1285 w1294 w1309 w1318 w1333 w1353 w1361 w1371 w1383 w1393 w1417 w1432 w1445 w1451 w1464 w1477 w1484 w1496 w1506 w1525 w1536 w1546 w1556 w1566 w1573 w1585 w1601 w1607 w1619 w1630] -> w212
      tunnel: w210 -> [w1141 w1150 w1163 w1181 w1191 w1202 w1213 w1225 w1237 w1247 w1256 w1269 w1284 w1302 w1311 w1317 w1339 w1352 w1360 w1370 w1382 w1392 w1408 w1431 w1442 w1450 w1463 w1476 w1487 w1495 w1517 w1527 w1533 w1543 w1553 w1563 w1575 w1587 w1598 w1609 w1621 w1632]
      tunnel: [w1141 w1150 w1163 w1181 w1191 w1202 w1213 w1225 w1237 w1247 w1256 w1269 w1284 w1302 w1311 w1317 w1338 w1352 w1360 w1370 w1382 w1392 w1407 w1431 w1442 w1450 w1463 w1476 w1487 w1495 w1517 w1527 w1533 w1543 w1553 w1563 w1575 w1587 w1597 w1609 w1621 w1632] -> w209
      tunnel: w207 -> [w1140 w1149 w1161 w1182 w1189 w1200 w1212 w1223 w1235 w1246 w1255 w1268 w1277 w1297 w1312 w1316 w1329 w1351 w1359 w1369 w1381 w1391 w1404 w1430 w1439 w1449 w1462 w1475 w1486 w1494 w1518 w1528 w1532 w1540 w1550 w1560 w1576 w1588 w1592 w1610 w1622 w1633]
      tunnel: [w1140 w1149 w1161 w1182 w1189 w1200 w1212 w1223 w1235 w1246 w1255 w1268 w1277 w1296 w1312 w1316 w1328 w1351 w1359 w1369 w1381 w1391 w1403 w1430 w1439 w1449 w1462 w1475 w1486 w1494 w1518 w1528 w1532 w1540 w1550 w1560 w1576 w1588 w1592 w1610 w1622 w1633] -> w206
      tunnel: w204 -> [w1137 w1148 w1162 w1183 w1190 w1201 w1211 w1224 w1236 w1245 w1254 w1267 w1276 w1293 w1313 w1315 w1325 w1348 w1358 w1368 w1380 w1390 w1401 w1428 w1438 w1448 w1461 w1474 w1485 w1493 w1519 w1529 w1531 w1539 w1549 w1559 w1577 w1589 w1591 w1604 w1616 w1627]
      tunnel: [w1137 w1148 w1162 w1183 w1190 w1201 w1211 w1224 w1236 w1245 w1254 w1267 w1276 w1293 w1313 w1315 w1325 w1348 w1358 w1368 w1380 w1390 w1400 w1428 w1438 w1448 w1461 w1474 w1485 w1493 w1519 w1529 w1531 w1539 w1549 w1559 w1577 w1589 w1591 w1604 w1614 w1626] -> w203
      tunnel: w201 -> [_ _ _ _ _ _ _ _ _ _ _ _ _ _ _ _ _ _ _ _ _ _ _ _ _ _ _ _ _ _ _ _ _ _ _ _ _ w1580 _ _ _ _]
      tunnel: [w1136 w1147 w1156 w1173 w1184 w1196 w1207 w1218 w1230 w1242 w1253 w1261 w1275 w1290 w1304 w1314 w1322 w1347 w1357 w1367 w1379 w1387 w1397 w1427 w1437 w1447 w1455 w1468 w1481 w1491 w1500 w1520 w1530 w1538 w1548 w1558 w1568 w1578 w1590 w1603 w1611 w1623] -> w197
      tunnel: w198 -> [w1136 w1147 w1156 w1173 w1184 w1196 w1207 w1218 w1230 w1242 w1253 w1261 w1275 w1290 w1305 w1314 w1322 w1347 w1357 w1367 w1379 w1387 w1397 w1427 w1437 w1447 w1455 w1468 w1481 w1491 w1500 w1520 w1530 w1538 w1548 w1558 w1568 w1578 w1590 w1603 w1611 w1623]
      frame "Exit" {
        # ">>State Logic  >>"
        # ">>> Time cluster >>>"
        # ">>> Yaw >>>"
        # ">>> Stepper position >>>"
        # ">>> Encoders >>>"
        # ">>> Object detection >>>"
        # ">>> Ultrasonic Sensors Detect >>>"
        n61 = call "Imaq Dispose"("All Images? (No)"=TRUE, "Image"=w1138) -> ()  [unwired: 4 in, 1 out]
      }
      frame "----Movement States----" {
        # ">>State Logic  >>"
        # ">>> Time cluster >>>"
        # ">>> Yaw >>>"
        # ">>> Stepper position >>>"
        # ">>> Encoders >>>"
        # ">>> Object detection >>>"
        # ">>> Ultrasonic Sensors Detect >>>"
      }
      frame "FORWARD" {
        # ">>State Logic  >>"
        # ">>> Time cluster >>>"
        # ">>> Yaw >>>"
        # ">>> Stepper position >>>"
        # ">>> Encoders >>>"
        # ">>> Object detection >>>"
        # ">>> Ultrasonic Sensors Detect >>>"
        n62 = Unbundle By Name(w1161) -> ("Yaw"=w1157:dbl)
        n63 = call "MOTOR CONTROL WITH PID AE.vi"("Yaw"=w1157, "Speed"=50.0, "Direction"=MOTOR_CONTROL_WITH_PID_AE_DIRECTION_TYPE_DEF."y-axis movement", "AE Mode"=MOTOR_CONTROL_WITH_PID_AE_DATA_MODE_TYPE_DEF."Write to AE") -> ()  [unwired: 1 out]
      }
      frame "FORWARD - IR ASSIST" {
        # ">>State Logic  >>"
        # ">>> Time cluster >>>"
        # ">>> Yaw >>>"
        # ">>> Stepper position >>>"
        # ">>> Encoders >>>"
        # ">>> Object detection >>>"
        # ">>> Ultrasonic Sensors Detect >>>"
        n64 = Unbundle By Name(w1173) -> ("Left IR Sensor"=w1172:dbl)
        n65 = Subtract(x=w1172, y=10.0) -> (x-y=w1170:dbl)
        n66 = Multiply(x=w1170, y=0.1) -> (x*y=w1168:dbl)
        n67 = call "MOTOR CONTROL WITH PID AE.vi"("Yaw"=w1168, "Speed"=40.0, "Direction"=MOTOR_CONTROL_WITH_PID_AE_DIRECTION_TYPE_DEF."y-axis movement", "AE Mode"=MOTOR_CONTROL_WITH_PID_AE_DATA_MODE_TYPE_DEF."Write to AE") -> ()  [unwired: 1 out]
      }
      frame "LEFT" {
        # ">>State Logic  >>"
        # ">>> Time cluster >>>"
        # ">>> Yaw >>>"
        # ">>> Stepper position >>>"
        # ">>> Encoders >>>"
        # ">>> Object detection >>>"
        # ">>> Ultrasonic Sensors Detect >>>"
        n68 = Unbundle By Name(w1189) -> ("Yaw"=w1186:dbl)
        n69 = call "MOTOR CONTROL WITH PID AE.vi"("Yaw"=w1186, "Speed"=-25.0, "Direction"=MOTOR_CONTROL_WITH_PID_AE_DIRECTION_TYPE_DEF."x-axis movement", "AE Mode"=MOTOR_CONTROL_WITH_PID_AE_DATA_MODE_TYPE_DEF."Write to AE") -> ()  [unwired: 1 out]
      }
      frame "R-ACW" {
        # ">>> IR Sensors >>>"
        # ">>> Time cluster >>>"
        # ">>> Yaw >>>"
        # ">>> Stepper position >>>"
        # ">>> Encoders >>>"
        # ">>> Object detection >>>"
        # ">>> Ultrasonic Sensors Detect >>>"
        n70 = call "MOTOR CONTROL WITH PID AE.vi"("Speed"=100.0, "Direction"=MOTOR_CONTROL_WITH_PID_AE_DIRECTION_TYPE_DEF."rotation", "AE Mode"=MOTOR_CONTROL_WITH_PID_AE_DATA_MODE_TYPE_DEF."Write to AE") -> ()  [unwired: 1 in, 1 out]
      }
      frame "R-CW" {
        (unwired) -0.2 ("Speed")
        # ">>> Time cluster >>>"
        # ">>> Yaw >>>"
        # ">>> Stepper position >>>"
        # ">>> Encoders >>>"
        # ">>> Object detection >>>"
        # ">>> Ultrasonic Sensors Detect >>>"
        n71 = call "MOTOR CONTROL WITH PID AE.vi"("Speed"=80.0, "Direction"=MOTOR_CONTROL_WITH_PID_AE_DIRECTION_TYPE_DEF."rotation", "AE Mode"=MOTOR_CONTROL_WITH_PID_AE_DATA_MODE_TYPE_DEF."Write to AE") -> ()  [unwired: 1 in, 1 out]
      }
      frame "RIGHT" {
        # ">>> Time cluster >>>"
        # ">>> Yaw >>>"
        # ">>> Stepper position >>>"
        # ">>> Encoders >>>"
        # ">>> Object detection >>>"
        # ">>> Ultrasonic Sensors Detect >>>"
        n72 = Unbundle By Name(w1223) -> ("Yaw"=w1219:dbl)
        n73 = call "MOTOR CONTROL WITH PID AE.vi"("Yaw"=w1219, "Speed"=50.0, "Direction"=MOTOR_CONTROL_WITH_PID_AE_DIRECTION_TYPE_DEF."x-axis movement", "AE Mode"=MOTOR_CONTROL_WITH_PID_AE_DATA_MODE_TYPE_DEF."Write to AE") -> ()  [unwired: 1 out]
      }
      frame "REVERSE" {
        # ">>> Time cluster >>>"
        # ">>> Yaw >>>"
        # ">>> Stepper position >>>"
        # ">>> Encoders >>>"
        # ">>> Object detection >>>"
        # ">>> Ultrasonic Sensors Detect >>>"
        n74 = Unbundle By Name(w1235) -> ("Yaw"=w1231:dbl)
        n75 = call "MOTOR CONTROL WITH PID AE.vi"("Yaw"=w1231, "Speed"=-50.0, "Direction"=MOTOR_CONTROL_WITH_PID_AE_DIRECTION_TYPE_DEF."y-axis movement", "AE Mode"=MOTOR_CONTROL_WITH_PID_AE_DATA_MODE_TYPE_DEF."Write to AE") -> ()  [unwired: 1 out]
      }
      frame "STOP" {
        n76 = Wait (ms)(milliseconds to wait=u32 100) -> ()  [unwired: 1 out]
        n77 = call "MOTOR CONTROL WITH PID AE.vi"("Direction"=MOTOR_CONTROL_WITH_PID_AE_DIRECTION_TYPE_DEF."stop", "AE Mode"=MOTOR_CONTROL_WITH_PID_AE_DATA_MODE_TYPE_DEF."Write to AE") -> ()  [unwired: 2 in, 1 out]
      }
      frame "----SENSOR READING---- " {
      }
      frame "READ ENCODERS" {
        # ">>> Time cluster >>>"
        # ">>> Yaw >>>"
        # ">>> Stepper position >>>"
        # ">>> Object detection >>>"
        # ">>> Current encoder distance >>>"
        # ">>> Ultrasonic Sensors Detect >>>"
        n78 = call "MOTOR CONTROL WITH PID AE.vi"("AE Mode"=MOTOR_CONTROL_WITH_PID_AE_DATA_MODE_TYPE_DEF."Read from AE") -> ("Speed & distance"=w1265:T1)  [unwired: 3 in]
        n79 = Unbundle By Name(w1265) -> ("xDistance"=w1264:dbl, "yDistance"=w1263:dbl, "wDistance"=w1262:dbl)
        n80 = Bundle By Name(cluster=w1272, "xDistance"=w1264, "yDistance"=w1263, "wDistance"=w1262) -> (w1271:T16)
      }
      frame "READ ULTRASONIC" {
        (unwired) navX_type_def."Read Values" ("Mode")
        (unwired) MOTOR_CONTROL_NO_PID_Type_Def."Latch" ("Direction")
        # ">>State Logic  >>"
        # ">>> Time cluster >>>"
        # ">>> Ultrasonic Sensors Detect >>>"
        # ">>> Object detection >>>"
        # ">>> Encoders >>>"
        # ">>> Stepper position >>>"
        # ">>> Yaw >>>"
        n81 = call "Arduino Interfacing VI.vi"("AE Mode"=Arduino_Interfacing."Read From Arduino") -> ("Arduino Data"=w1282:T4)  [unwired: 3 in, 1 out]
        n82 = Unbundle By Name(w1282) -> ("PING A"=w1281:u8, "PING B"=w1280:u8, "PING C"=w1279:u8, "PING D"=w1278:u8)
        n83 = Bundle By Name(cluster=w1288, "PING_A"=w1281, "PING_B"=w1280, "PING_C"=w1279, "PING_D"=w1278) -> (w1289:T15)
      }
      frame "READ YAW" {
        # ">>> Time cluster >>>"
        # ">>> Yaw >>>"
        # ">>> Ultrasonic Sensors Detect >>>"
        # ">>> Object detection >>>"
        # ">>> Encoders >>>"
        # ">>> Stepper position >>>"
        n84 = call "navX reading VI.vi"("Mode"=navX_type_def."Read Values") -> ("NavX Readings"=w1292:T3)  [unwired: 2 in, 3 out]
        n85 = Unbundle By Name(w1292) -> ("Heading"=w1291:dbl)
        n86 = Unbundle By Name(w1292) -> ("Yaw"=w1295:dbl)
        n87 = Bundle By Name(cluster=w1297, "Yaw"=w1295, "Compass"=w1291) -> (w1296:T11)
      }
      frame "READ IR" {
        w1307 = T33 [enum."A/AI0"] items=["Not Connected", "AudioIn/Left", "AudioIn/Right", "C/AI0", "C/AI1", "A/AI0", "A/AI1", "A/AI2", "A/AI3", "A/AI4", "A/AI5", "A/AI6", "A/AI7", "B/AI0", "B/AI1", "B/AI2", "B/AI3", "B/AI4", "B/AI5", "B/AI6", "B/AI7", "AI/AI0", "AI/AI1", "AI/AI2", "AI/AI3", "A/AI0 (DIFF)", "A/AI1 (DIFF)", "A/AI2 (DIFF)", "A/AI3 (DIFF)", "B/AI0 (DIFF)", "B/AI1 (DIFF)", "B/AI2 (DIFF)", "B/AI3 (DIFF)"] ("AI Channel")
        # ">>State Logic  >>"
        # ">>> Time cluster >>>"
        # ">>> Ultrasonic Sensors Detect >>>"
        # ">>> Object detection >>>"
        # ">>> Encoders >>>"
        # ">>> Stepper position >>>"
        # ">>> Yaw >>>"
        n88 = call <vilib>:"Sharp IR.vi"("AI Channel"=w1307) -> ("Sharp IR Distance"=w1303:dbl)  [unwired: 8 in, 2 out]
        n89 = Bundle By Name(cluster=w1305, "Left IR Sensor"=w1303) -> (w1304:T8)
      }
      frame "----SYSTEM MODES----" {
        (unwired) I2C_MASTER_Type_Def."Last State" ("Arduino Mode")
        # ">>> Object detection >>>"
        # ">>> Yaw >>>"
        # ">>> Ultrasonic Sensors Detect >>>"
        # ">>> Encoders >>>"
        # ">>> Stepper position >>>"
      }
      frame "INIT" {
        w1340 = u8 0
        w1341 = 0.0
        # ">>> Time cluster >>>"
        # ">>> Object detection >>>"
        # ">>> Yaw >>>"
        # ">>> Ultrasonic Sensors Detect >>>"
        # ">>> Encoders >>>"
        # ">>> Stepper position >>>"
        # ">>State Logic  >>"
        n90 = call "Arduino Interfacing VI.vi"("AE Mode"=Arduino_Interfacing."Initialize") -> ()  [unwired: 3 in, 2 out]
        n91 = call "FGV Bool.vi"("Init/Read/Write State"=States_for_Action_Engine."Initialize") -> ()  [unwired: 2 in, 2 out]
        n92 = call "Elasped Timer.vi"("Action"=Elapsed_timer_control."Initialize") -> ()  [unwired: 7 in, 4 out]
        n93 = call "MOTOR CONTROL WITH PID AE.vi"("AE Mode"=MOTOR_CONTROL_WITH_PID_AE_DATA_MODE_TYPE_DEF."Init AE") -> ()  [unwired: 3 in, 1 out]
        n94 = Bundle By Name(cluster=w1334, "Recognized Object"=FALSE, "Object X coordinate"=0.0, "Object Y coordinate"=0.0) -> (w1333:T14)
        n95 = Bundle By Name(cluster=w1339, "y Stepper Position"=u8 0, "z Stepper Position"=u8 0) -> (w1338:T12)
        n96 = Bundle By Name(cluster=w1343, "xDistance"=w1341, "yDistance"=w1341, "wDistance"=w1341) -> (w1342:T16)
        n97 = Bundle By Name(cluster=w1345, "PING_A"=w1340, "PING_B"=w1340, "PING_C"=w1340, "PING_D"=w1340) -> (w1346:T15)
        n98 = Bundle By Name(cluster=w1329, "Yaw"=0.0) -> (w1328:T11)
      }
      frame "ARDUINO - ULTRASONIC" {
        # ">>> Object detection >>>"
        # ">>> Yaw >>>"
        # ">>> Ultrasonic Sensors Detect >>>"
        # ">>> Encoders >>>"
        # ">>> Stepper position >>>"
        # ">>State Logic  >>"
        n99 = call "Arduino Interfacing VI.vi"("Data to Write"=I2C_MASTER_WRITE_NEW_Type_Def."Ultrasonic sensors", "AE Mode"=Arduino_Interfacing."Write to Arduino") -> ()  [unwired: 2 in, 2 out]
      }
      frame "NAVX CALIBRATE" {
        # ">>> Object detection >>>"
        # ">>> Yaw >>>"
        # ">>> Ultrasonic Sensors Detect >>>"
        # ">>> Encoders >>>"
        # ">>> Stepper position >>>"
        # ">>State Logic  >>"
        # "Adds a 15 second delay to the startup process \nfor the NavX to calibrate"
        n100 = Wait (ms)(milliseconds to wait=u32 5000) -> ()  [unwired: 1 out]
      }
      frame "NO ACTION", Default {
        (unwired) u8 0 ("y Stepper value")
        (unwired) TRUE ("Latch")
        (unwired) navX_type_def."Read Values" ("Mode")
        (unwired) MOTOR_CONTROL_NO_PID_Type_Def."Latch" ("Direction")
        # ">>> Object detection >>>"
        # ">>> Yaw >>>"
        # ">>> Ultrasonic Sensors Detect >>>"
        # ">>> Encoders >>>"
        # ">>> Stepper position >>>"
        # ">>State Logic  >>"
        n101 = case shown="4" w1373 {
          tunnel: [0 100] -> w1375
          frame 1, Default {
          }
          frame 4 {
          }
        }
      }
      frame "----RESET CASES----" {
        (unwired) I2C_MASTER_Type_Def."Last State" ("Arduino Mode")
        # ">>> Object detection >>>"
        # ">>> Yaw >>>"
        # ">>> Ultrasonic Sensors Detect >>>"
        # ">>> Encoders >>>"
        # ">>> Stepper position >>>"
        # ">>State Logic  >>"
      }
      frame "RESET ENCODERS" {
        # ">>> Object detection >>>"
        # ">>> Yaw >>>"
        # ">>> Ultrasonic Sensors Detect >>>"
        # ">>> Encoders >>>"
        # ">>> Stepper position >>>"
        # ">>State Logic  >>"
        n102 = call "MOTOR CONTROL WITH PID AE.vi"("Direction"=MOTOR_CONTROL_WITH_PID_AE_DIRECTION_TYPE_DEF."reset encoders", "AE Mode"=MOTOR_CONTROL_WITH_PID_AE_DATA_MODE_TYPE_DEF."Write to AE") -> ()  [unwired: 2 in, 1 out]
      }
      frame "RESET FLAGS" {
        (unwired) I2C_MASTER_Type_Def."Last State" ("Arduino Mode")
        # "Resets any software variables\nand/or non-critical states"
        n103 = Wait (ms)(milliseconds to wait=u32 20) -> ()  [unwired: 1 out]
        n104 = Bundle By Name(cluster=w1401, "Time up flag"=FALSE, "SET TIME TO CHECK"=0.0) -> (w1400:T10)
        n105 = Bundle By Name(cluster=w1418, "Recognized Object"=FALSE, "Object X coordinate"=0.0, "Object Y coordinate"=0.0) -> (w1417:T14)
        n106 = Bundle By Name(cluster=w1408, "y Stepper Position"=u8 0, "z Stepper Position"=u8 0) -> (w1407:T12)
        n107 = Bundle By Name(cluster=w1413, "xDistance"=0.0, "yDistance"=0.0, "wDistance"=0.0) -> (w1412:T16)
        n108 = Bundle By Name(cluster=w1425, "PING_A"=u8 0, "PING_B"=u8 0, "PING_C"=u8 0, "PING_D"=u8 0) -> (w1424:T15)
        n109 = Bundle By Name(cluster=w1404, "Yaw"=0.0) -> (w1403:T11)
      }
      frame "RESET YAW" {
        n110 = Wait (ms)(milliseconds to wait=u32 100) -> ()  [unwired: 1 out]
        n111 = call "navX reading VI.vi"("Mode"=navX_type_def."Zero Yaw") -> ()  [unwired: 2 in, 4 out]
      }
      frame "RESET ARM" {
        n112 = call "Arduino Interfacing VI.vi"("Data to Write"=I2C_MASTER_WRITE_NEW_Type_Def."Soft Reset", "AE Mode"=Arduino_Interfacing."Write to Arduino") -> ()  [unwired: 2 in, 2 out]
      }
      frame "--------CAM STATES-------" {
      }
      frame "OPEN LOG CAM" {
        n113 = call "Webcam AE.vi"("Session In"=T30 "cam0", "Camera states"=Webcam_AE."Initialize Camera") -> ("error out"=w1458:errorcluster, "Session Out"=w1457:T30)  [unwired: 1 in, 1 out]
        n114 = call "Webcam AE.vi"("error in (no error)"=w1458, "Session In"=w1457, "Camera states"=Webcam_AE."Open Camera") -> ()  [unwired: 3 out]
      }
      frame "OPEN LIFE CAM" {
        n115 = call "Webcam AE.vi"("Session In"=T30 "cam1", "Camera states"=Webcam_AE."Initialize Camera") -> ("error out"=w1471:errorcluster, "Session Out"=w1470:T30)  [unwired: 1 in, 1 out]
        n116 = call "Webcam AE.vi"("error in (no error)"=w1471, "Session In"=w1470, "Camera states"=Webcam_AE."Open Camera") -> ()  [unwired: 3 out]
      }
      frame "CAM ACQ" {
        # ">>State Logic  >>"
        # ">>> Time cluster >>>"
        # ">>> Yaw >>>"
        # ">>> Stepper position >>>"
        # ">>> Encoders >>>"
        # ">>> Object detection >>>"
        # ">>> Ultrasonic Sensors Detect >>>"
        n117 = call "Webcam AE.vi"("error in (no error)"=w1482, "Camera states"=Webcam_AE."Continuous Acquisition") -> ()  [unwired: 1 in, 3 out]
      }
      frame "CAM CLOSE" {
        # ">>State Logic  >>"
        # ">>> Time cluster >>>"
        # ">>> Yaw >>>"
        # ">>> Stepper position >>>"
        # ">>> Encoders >>>"
        # ">>> Object detection >>>"
        # ">>> Ultrasonic Sensors Detect >>>"
        n118 = call "Webcam AE.vi"("Camera states"=Webcam_AE."Close Camera") -> ()  [unwired: 2 in, 3 out]
      }
      frame "PROCESS IMAGE" {
        # ">>State Logic  >>"
        # ">>> Time cluster >>>"
        # ">>> Yaw >>>"
        # ">>> Stepper position >>>"
        # ">>> Encoders >>>"
        # ">>> Object detection >>>"
        # ">>> Ultrasonic Sensors Detect >>>"
        n119 = call "Webcam AE.vi"("error in (no error)"=w1512, "Camera states"=Webcam_AE."Retrieve Image") -> ("error out"=w1508:errorcluster, "Image Out"=w1511:T23)  [unwired: 1 in, 1 out]
        n120 = call "Object Detection SubVI.vi"("Error In"=w1508, "Mode"="Object recognition mode", "Image Dest"=w1510, "Image in"=w1511) -> ("Object Center Coordinates"=w1505:cluster{"x":sgl, "y":sgl}, "Object detection cluster"=w1501:T2)  [unwired: 2 out]
        "Object detection cluster" <- w1501
        "Object Center Coordinates" <- w1505
        n121 = Unbundle By Name(w1501) -> ("Object detected?"=w1502:bool)
        n122 = Unbundle By Name(w1505) -> ("x"=w1504:sgl, "y"=w1503:sgl)
        n123 = Bundle By Name(cluster=w1507, "Recognized Object"=w1502, "Object X coordinate"=w1504, "Object Y coordinate"=w1503) -> (w1506:T14)
      }
      frame "DISPOSE BUFFERS" {
        # ">>State Logic  >>"
        # ">>> Time cluster >>>"
        # ">>> Yaw >>>"
        # ">>> Stepper position >>>"
        # ">>> Encoders >>>"
        # ">>> Object detection >>>"
        # ">>> Ultrasonic Sensors Detect >>>"
        n124 = call "Webcam AE.vi"("error in (no error)"=w1522, "Camera states"=Webcam_AE."Dispose Image Buffers") -> ()  [unwired: 1 in, 3 out]
      }
      frame "-----ARM ACTIONS-----" {
      }
      frame "CLOSE CLAW" {
        n125 = call "Arduino Interfacing VI.vi"("Data to Write"=I2C_MASTER_WRITE_NEW_Type_Def."Close Claw", "AE Mode"=Arduino_Interfacing."Write to Arduino") -> ()  [unwired: 2 in, 2 out]
      }
      frame "OPEN CLAW" {
        n126 = call "Arduino Interfacing VI.vi"("Data to Write"=I2C_MASTER_WRITE_NEW_Type_Def."Open Claw", "AE Mode"=Arduino_Interfacing."Write to Arduino") -> ()  [unwired: 2 in, 2 out]
      }
      frame "Z STEPPER CAM HEIGHT" {
        n127 = call "Arduino Interfacing VI.vi"("Data to Write"=I2C_MASTER_WRITE_NEW_Type_Def."zStepper 8k", "AE Mode"=Arduino_Interfacing."Write to Arduino") -> ()  [unwired: 2 in, 2 out]
      }
      frame "Z STEPPER GRAB HEIGHT" {
        # ">>State Logic  >>"
        # ">>> Time cluster >>>"
        # ">>> Yaw >>>"
        # ">>> Stepper position >>>"
        # ">>> Encoders >>>"
        # ">>> Object detection >>>"
        # ">>> Ultrasonic Sensors Detect >>>"
        n128 = call "Arduino Interfacing VI.vi"("Data to Write"=I2C_MASTER_WRITE_NEW_Type_Def."zStepper 100", "AE Mode"=Arduino_Interfacing."Write to Arduino") -> ()  [unwired: 2 in, 2 out]
      }
      frame "Y STEPPER CONTROL" {
        # ">>State Logic  >>"
        # ">>> yStepper command>>>"
        # ">>> Time cluster >>>"
        # ">>> Yaw >>>"
        # ">>> Stepper position >>>"
        # ">>> Encoders >>>"
        # ">>> Object detection >>>"
        # ">>> Ultrasonic Sensors Detect >>>"
        n129 = Unbundle By Name(w1580) -> ("yStepper desired"=w1579:u8)
        n130 = call "Arduino Interfacing VI.vi"("y Stepper value"=w1579, "Data to Write"=I2C_MASTER_WRITE_NEW_Type_Def."yStepper control", "AE Mode"=Arduino_Interfacing."Write to Arduino") -> ()  [unwired: 1 in, 2 out]
      }
      frame "READ STEPPER VALUES" {
        # ">>State Logic  >>"
        # ">>> Time cluster >>>"
        # ">>> Yaw >>>"
        # ">>> Stepper position >>>"
        # ">>> Encoders >>>"
        # ">>> Object detection >>>"
        # ">>> Ultrasonic Sensors Detect >>>"
        n131 = call "Arduino Interfacing VI.vi"("AE Mode"=Arduino_Interfacing."Read From Arduino") -> ("Arduino Data"=w1595:T4)  [unwired: 3 in, 1 out]
        n132 = Unbundle By Name(w1595) -> ("y Stepper Position"=w1594:u8, "z Stepper Position"=w1593:u8)
        n133 = Bundle By Name(cluster=w1598, "y Stepper Position"=w1594, "z Stepper Position"=w1593) -> (w1597:T12)
      }
      frame " -----TIMING-----" {
        # ">>State Logic  >>"
        # ">>> Time cluster >>>"
        # ">>> Yaw >>>"
        # ">>> Stepper position >>>"
        # ">>> Encoders >>>"
        # ">>> Object detection >>>"
        # ">>> Ultrasonic Sensors Detect >>>"
      }
      frame "SET TIMER" {
        # ">>State Logic  >>"
        # ">>> Time cluster >>>"
        # ">>> Yaw >>>"
        # ">>> Stepper position >>>"
        # ">>> Encoders >>>"
        # ">>> Object detection >>>"
        # ">>> Ultrasonic Sensors Detect >>>"
        n134 = call "Elasped Timer.vi"("Time Setting"=5.0, "Action"=Elapsed_timer_control."Initialize") -> ()  [unwired: 6 in, 4 out]
        n135 = Bundle By Name(cluster=w1616, "Time up flag"=FALSE) -> (w1614:T10)
      }
      frame "START TIMER" {
        # ">>State Logic  >>"
        # ">>> Time cluster >>>"
        # ">>> Yaw >>>"
        # ">>> Stepper position >>>"
        # ">>> Encoders >>>"
        # ">>> Object detection >>>"
        # ">>> Ultrasonic Sensors Detect >>>"
        n136 = call "Elasped Timer.vi"("Action"=Elapsed_timer_control."Start") -> ("Time Out?!"=w1624:bool)  [unwired: 7 in, 3 out]
        n137 = Bundle By Name(cluster=w1627, "Time up flag"=w1624) -> (w1626:T10)
      }
    }
    "State Logic" <- w225
    n138 = local read "TASK ENABLE"() -> (w219:bool)
    n139 = Not(x=w219) -> (.not. x?=w218:bool)
    n140 = case shown="True" w226 {
      tunnel: w230 -> [w254 w287]
      tunnel: w234 -> [w250 w289]
      tunnel: [w254 w287] -> w239
      tunnel: [w250 w290] -> w238
      tunnel: w235 -> [_ w285]
      tunnel: w237 -> [_ w286]
      tunnel: w232 -> [w253 w292]
      tunnel: [w253 w292] -> w231
      tunnel: "STOP TASK" -> [_ w275]
      tunnel: w225 -> [w252 w291]
      tunnel: [w252 w288] -> w224
      tunnel: w221 -> [w251 w281]
      tunnel: [w251 w281] -> w220
      tunnel: w218 -> [_ w276]
      tunnel: [w249 w273] -> w217
      tunnel: w216 -> [w249 w272]
      tunnel: w212 -> [w248 w269]
      tunnel: [w248 w269] -> w211
      tunnel: w209 -> [w247 w265]
      tunnel: [w247 w265] -> w208
      tunnel: w206 -> [w246 w263]
      tunnel: [w246 w263] -> w205
      tunnel: w203 -> [w245 w261]
      tunnel: [w245 w261] -> w202
      tunnel: w201 -> [w244 w260]
      tunnel: [w244 w259] -> w200
      tunnel: [_ w257] -> w199
      tunnel: w197 -> [w243 w255]
      tunnel: [w243 w255] -> w196
      frame False {
        # ">>> IR Sensors >>>"
        # ">>> IR Sensors >>>"
        # ">>> yStepper command>>>"
        # ">>> Time cluster >>>"
        # ">>> Yaw >>>"
        # ">>> Stepper position >>>"
        # ">>> Encoders >>>"
        # ">>> Object detection >>>"
        # ">>> Ultrasonic Sensors Detect >>>"
        # ">>> Time cluster >>>"
        # ">>> Yaw >>>"
        # ">>> Stepper position >>>"
        # ">>> Encoders >>>"
        # ">>> Object detection >>>"
        # ">>> Ultrasonic Sensors Detect >>>"
      }
      frame True {
        # ">>State Logic Queue Reference >>"
        # ">>Timeout>>"
        # ">>> yStepper command>>>"
        # ">>> Time cluster >>>"
        # ">>> Object detection >>>"
        # ">>> Yaw >>>"
        # ">>> Ultrasonic Sensors Detect >>>"
        # ">>> Encoders >>>"
        # ">>> Stepper position >>>"
        # ">>State Logic  >>"
        # ">>True Stop Next State >>"
        # ">>Action Queue>>"
        # ">> Manual override >>"
        # ">>> Time cluster >>>"
        # ">>> Yaw >>>"
        # ">>> Stepper position >>>"
        # ">>> Encoders >>>"
        # ">>> Object detection >>>"
        # ">>> Ultrasonic Sensors Detect >>>"
        # ">>Action Queue>>"
        # ">>State Logic Queue Reference >>"
        n141 = Or(x=w275, y=w276) -> (x .or. y?=w274:bool)
        n142 = Unbundle By Name(w255) -> ("Left IR Sensor"=w256:dbl)
        "Left IR Sensor" <- w256
        n143 = Unbundle By Name(w261) -> ("Time up flag"=w262:bool)
        "Time up flag" <- w262
        n144 = Unbundle By Name(w263) -> ("Yaw"=w264:dbl, "Compass"=w258:dbl)
        n145 = Unbundle By Name(w265) -> ("y Stepper Position"=w267:u8, "z Stepper Position"=w266:u8)
        n146 = Unbundle By Name(w281) -> ("xDistance"=w278:dbl, "yDistance"=w279:dbl, "wDistance"=w280:dbl)
        n147 = Unbundle By Name(w269) -> ("Recognized Object"=w268:bool, "Object X coordinate"=w271:dbl, "Object Y coordinate"=w270:dbl)
        n148 = Unbundle By Name(w292) -> ("PING_A"=w284:u8, "PING_B"=w283:u8, "PING_C"=w282:u8, "PING_D"=w277:u8)
        n149 = case shown="33" w291 {
          tunnel: [w295 w301 w313 w322 w389 w402 w437 w489 w529 w571 w623 w669 w708 w767 w811 w850 w895 w938 w980 w1010 w1057 w1097] -> w290
          tunnel: w289 -> [w295 w304 w314 w325 w391 w403 w446 w487 w530 w577 w616 w672 w715 w757 w814 w856 w894 w933 w971 w1014 w1064 w1102]
          tunnel: [State_Type_Definitions."Idle" ("Enum") State_Type_Definitions."Idle" ("Enum") w309 w324 State_Type_Definitions."Shutdown" ("Enum") w404 w444 w490 w528 w572 w622 w670 w710 w766 w812 w857 w896 w939 w972 w1011 w1058 w1098] -> w288
          tunnel: w287 -> [_ _ w312 w328 _ w409 w440 w486 w537 w576 w620 w673 w714 w764 w809 w855 w892 w936 w979 w1018 w1063 w1105]
          tunnel: w286 -> [_ _ _ w327 _ w408 w439 w485 w536 w575 w619 w666 w713 w763 w808 w854 w891 w935 w977 w1013 w1062 w1104]
          tunnel: w285 -> [_ _ w311 w323 _ w407 w438 w484 w535 w574 w618 w665 w712 w765 w810 w853 w890 w934 w978 w1017 w1061 w1103]
          tunnel: w274 -> [_ _ _ _ _ w401 w445 w483 w532 w570 w621 w671 w716 w758 w815 w851 w893 w937 w975 w1016 w1056 w1101]
          tunnel: w284 -> [_ _ _ _ _ _ _ _ _ _ _ _ _ _ _ _ _ _ _ _ _ _]
          tunnel: w283 -> [_ _ _ _ _ _ _ w482 _ _ w612 w654 w706 _ w801 _ _ _ _ _ _ _]
          tunnel: w282 -> [_ _ _ _ _ _ _ w481 _ _ w613 w655 w707 _ w802 _ _ _ _ _ _ _]
          tunnel: w280 -> [_ _ _ _ _ _ _ _ w534 _ _ _ _ _ _ _ _ _ _ _ _ _]
          tunnel: w279 -> [_ _ _ _ _ w400 _ _ _ _ _ _ w711 _ _ _ _ _ _ _ _ _]
          tunnel: w278 -> [_ _ _ _ _ _ _ _ _ _ _ w660 _ _ _ _ _ _ _ _ _ _]
          tunnel: w277 -> [_ _ _ _ _ _ _ _ _ _ _ _ _ _ _ _ _ _ _ _ _ _]
          tunnel: [State_Type_Definitions."Idle" ("Enum") State_Type_Definitions."Idle" ("Enum") State_Type_Definitions."Idle" ("Enum") State_Type_Definitions."Idle" ("Enum") State_Type_Definitions."Shutdown" ("Enum") w397 w443 w488 w525 w569 w615 w668 w709 w768 w813 w849 w897 w940 w973 w1012 w1059 w1100] -> w273
          tunnel: w272 -> [_ _ w309 _ _ _ _ _ _ _ _ _ _ _ _ _ _ _ _ _ _ _]
          tunnel: w268 -> [_ _ _ _ _ _ _ _ _ _ _ _ _ _ _ _ w887 _ w974 _ _ _]
          tunnel: w271 -> [_ _ _ _ _ _ _ _ _ _ _ _ _ _ _ _ _ _ _ _ _ _]
          tunnel: w270 -> [_ _ _ _ _ _ _ _ _ _ _ _ _ _ _ _ _ _ _ _ _ _]
          tunnel: w267 -> [_ _ _ _ _ _ _ _ _ _ _ _ _ _ _ _ _ _ _ _ _ _]
          tunnel: w266 -> [_ _ _ _ _ _ w442 _ _ w567 _ _ _ w761 _ _ _ w932 _ w1015 _ _]
          tunnel: w264 -> [_ _ _ _ _ _ _ _ _ _ _ _ _ _ _ _ _ _ _ _ _ _]
          tunnel: w262 -> [_ _ _ _ _ _ _ _ _ _ _ _ _ _ _ w847 _ _ _ _ _ _]
          tunnel: w260 -> [w293 w299 w308 w320 w387 w396 w441 w480 w524 w568 w614 w664 w705 w756 w806 w848 w888 w929 w970 w1009 w1060 w1099]
          tunnel: [w293 w298 w308 w320 w387 w396 w441 w480 w524 w568 w614 w664 w705 w756 w806 w848 w888 w929 w970 w1009 w1060 w1099] -> w259
          tunnel: w258 -> [_ _ _ _ _ _ _ _ _ _ _ _ _ _ _ _ _ _ _ _ w1055 _]
          tunnel: [_ _ _ TRUE _ _ _ _ _ _ _ _ _ _ _ _ _ _ _ _ _ _] -> w257
          tunnel: w256 -> [_ _ _ _ _ _ _ _ _ _ _ _ _ _ _ _ _ _ _ _ _ _]
          frame 0 {
            # ">>> yStepper command>>>"
          }
          frame 1 {
            # ">>> yStepper command>>>"
            n150 = for {
              shift-right: [w307] -> w301
              shift-left: w304 -> [w306]
              tunnel: string[] ["INIT", "RESET ARM", "RESET FLAGS", "RESET YAW", "NAVX CALIBRATE"] -> [w305] mode=indexing
              n151 = Enqueue Element(queue=w306, element=w305) -> (queue out=w307:refnum<queue>)  [unwired: 2 in, 2 out]
            }
            n152 = Bundle By Name(cluster=w299, "yStepper desired"=u8 0) -> (w298:T9)
          }
          frame 3 {
            # ">>> yStepper command>>>"
            n153 = Flush Queue(queue=w312, error in (no error)=w311) -> ()  [unwired: 3 out]
            n154 = for {
              shift-right: [w318] -> w313
              shift-left: w314 -> [w317]
              tunnel: string[] ["STOP", "RESET ENCODERS", "RESET YAW", "RESET ARM", "RESET FLAGS", "DISPOSE BUFFERS", "CAM CLOSE"] -> [w316] mode=indexing
              n155 = Enqueue Element(queue=w317, element=w316) -> (queue out=w318:refnum<queue>)  [unwired: 2 in, 2 out]
            }
          }
          frame 4, Default {
            (unwired) TRUE ("Green LED")
            # ">>> yStepper command>>>"
            n156 = Dequeue Element(queue=w328, timeout in ms (-1)=w327, error in (no error)=w323) -> (element=w326:T7)  [unwired: 3 out]
            n157 = case shown="\"Start Task 9\"" w326 {
              tunnel: [w330 w337 w344 w351 w358 w365 w372 w374 w382] -> w322
              tunnel: w325 -> [w331 w338 w345 w352 w359 w366 w372 w375 w381]
              tunnel: [State_Type_Definitions."Task 1" ("Enum") State_Type_Definitions."Task 2:Raise Arm" ("Enum") State_Type_Definitions."Task 3" ("Enum") State_Type_Definitions."Task 4_A" ("Enum") State_Type_Definitions."Task 5_A" ("Enum") State_Type_Definitions."Task 6_A" ("Enum") State_Type_Definitions."Idle" ("Enum") State_Type_Definitions."Shutdown" ("Enum") State_Type_Definitions."Task 9A: Raise Arm" ("Enum")] -> w324
              frame "Start Task 1" {
                n158 = for {
                  shift-right: [w335] -> w330
                  shift-left: w331 -> [w334]
                  tunnel: string[] ["RESET ENCODERS", "RESET YAW", "FORWARD", "READ ENCODERS"] -> [w333] mode=indexing
                  n159 = Enqueue Element(queue=w334, element=w333) -> (queue out=w335:refnum<queue>)  [unwired: 2 in, 2 out]
                }
              }
              frame "Start Task 2" {
                n160 = for {
                  shift-right: [w342] -> w337
                  shift-left: w338 -> [w341]
                  tunnel: string[] ["RESET ENCODERS", "RESET YAW", "READ ULTRASONIC", "ARDUINO - ULTRASONIC"] -> [w340] mode=indexing
                  n161 = Enqueue Element(queue=w341, element=w340) -> (queue out=w342:refnum<queue>)  [unwired: 2 in, 2 out]
                }
              }
              frame "Start Task 3" {
                n162 = for {
                  shift-right: [w349] -> w344
                  shift-left: w345 -> [w348]
                  tunnel: string[] ["RESET ENCODERS", "READ ENCODERS", "R-ACW"] -> [w347] mode=indexing
                  n163 = Enqueue Element(queue=w348, element=w347) -> (queue out=w349:refnum<queue>)  [unwired: 2 in, 2 out]
                }
              }
              frame "Start Task 4" {
                n164 = for {
                  shift-right: [w356] -> w351
                  shift-left: w352 -> [w355]
                  tunnel: string[] ["RESET YAW", "RESET ENCODERS", "RESET ARM", "RESET FLAGS", "", ""] -> [w354] mode=indexing
                  n165 = Enqueue Element(queue=w355, element=w354) -> (queue out=w356:refnum<queue>)  [unwired: 2 in, 2 out]
                }
              }
              frame "Start Task 5" {
                n166 = for {
                  shift-right: [w363] -> w358
                  shift-left: w359 -> [w362]
                  tunnel: string[] ["RESET YAW", "RESET ENCODERS", "READ STEPPER VALUES", "Z STEPPER CAM HEIGHT", "", ""] -> [w361] mode=indexing
                  n167 = Enqueue Element(queue=w362, element=w361) -> (queue out=w363:refnum<queue>)  [unwired: 2 in, 2 out]
                }
              }
              frame "Start Task 6" {
                n168 = for {
                  shift-right: [w370] -> w365
                  shift-left: w366 -> [w369]
                  tunnel: string[] ["OPEN LOG CAM ", "", "", "", "", ""] -> [w368] mode=indexing
                  n169 = Enqueue Element(queue=w369, element=w368) -> (queue out=w370:refnum<queue>)  [unwired: 2 in, 2 out]
                }
              }
              frame "None", Default {
              }
              frame "Exit" {
                n170 = for {
                  shift-right: [w379] -> w374
                  shift-left: w375 -> [w378]
                  tunnel: string[] ["STOP", "RESET ENCODERS", "RESET YAW", "EXIT"] -> [w377] mode=indexing
                  n171 = Enqueue Element(queue=w378, element=w377) -> (queue out=w379:refnum<queue>)  [unwired: 2 in, 2 out]
                }
              }
              frame "Start Task 9" {
                n172 = for {
                  shift-right: [w386] -> w382
                  shift-left: w381 -> [w385]
                  tunnel: string[] ["RESET ENCODERS", "READ ENCODERS", "Z STEPPER CAM HEIGHT"] -> [w384] mode=indexing
                  n173 = Enqueue Element(queue=w385, element=w384) -> (queue out=w386:refnum<queue>)  [unwired: 2 in, 2 out]
                }
              }
            }
          }
          frame 5 {
            # ">>> yStepper command>>>"
            n174 = for {
              shift-right: [w395] -> w389
              shift-left: w391 -> [w394]
              tunnel: string[] ["INIT", "RESET ENCODERS", "RESET FLAGS", "CAM CLOSE", "DISPOSE BUFFERS", "EXIT", ""] -> [w393] mode=indexing
              n175 = Enqueue Element(queue=w394, element=w393) -> (queue out=w395:refnum<queue>)  [unwired: 2 in, 2 out]
            }
          }
          frame 6 {
            # ">>> yStepper command>>>"
            # "Use 250"
            n176 = Dequeue Element(queue=w409, timeout in ms (-1)=w408, error in (no error)=w407) -> (element=w406:T7)  [unwired: 3 out]
            n177 = Greater?(x=w400, y=250.0) -> (0:w398:bool)
            n178 = Or(x=w398, y=w401) -> (x .or. y?=w405:bool)
            n179 = case shown="\"None\", Default" w406 {
              tunnel: w405 -> [w412 _]
              tunnel: [w416 State_Type_Definitions."True Stop" ("Enum")] -> w404
              tunnel: w403 -> [w413 w431]
              tunnel: [w411 w430] -> w402
              tunnel: [State_Type_Definitions."Idle" ("Enum") State_Type_Definitions."Shutdown" ("Enum")] -> w397
              frame "None", Default {
                n180 = case shown="True" w412 {
                  tunnel: w413 -> [w419 w425]
                  tunnel: [w418 w423] -> w411
                  frame False {
                    n181 = for {
                      shift-right: [w421] -> w418
                      shift-left: w419 -> [w422]
                      tunnel: string[] ["READ ENCODERS", "READ YAW", "FORWARD"] ("element") -> [w420] mode=indexing
                      n182 = Enqueue Element(queue=w422, element=w420) -> (queue out=w421:refnum<queue>)  [unwired: 2 in, 2 out]
                    }
                  }
                  frame True {
                    n183 = for {
                      shift-right: [w427] -> w423
                      shift-left: w425 -> [w428]
                      tunnel: string[] ["RESET YAW", "RESET ENCODERS", "STOP", ""] -> [w426] mode=indexing
                      n184 = Enqueue Element(queue=w428, element=w426) -> (queue out=w427:refnum<queue>)  [unwired: 2 in, 2 out]
                    }
                  }
                }
                n185 = Select(t=State_Type_Definitions."True Stop" ("Enum"), s=w412, f=State_Type_Definitions."Task 1" ("Enum")) -> (s? t:f=w416:u16)
              }
              frame "Exit" {
                n186 = for {
                  shift-right: [w435] -> w430
                  shift-left: w431 -> [w436]
                  tunnel: string[] ["STOP", "RESET ENCODERS", "RESET YAW", ""] -> [w434] mode=indexing
                  n187 = Enqueue Element(queue=w436, element=w434) -> (queue out=w435:refnum<queue>)  [unwired: 2 in, 2 out]
                }
              }
            }
          }
          frame 8 {
            # ">> Stepper height reeached >>"
            # ">>> yStepper command>>>"
            # ">> Manual override >>"
            n188 = Dequeue Element(queue=w440, timeout in ms (-1)=w439, error in (no error)=w438) -> (element=w449:T7)  [unwired: 3 out]
            n189 = Equal?(x=w442, y=u8 80) -> (x = y?=w447:bool)
            n190 = case shown="\"None\", Default" w449 {
              tunnel: [w460 State_Type_Definitions."True Stop" ("Enum")] -> w444
              tunnel: [w458 w475] -> w437
              tunnel: w446 -> [w457 _]
              tunnel: w445 -> [w451 _]
              tunnel: [State_Type_Definitions."Idle" ("Enum") State_Type_Definitions."Shutdown" ("Enum")] -> w443
              tunnel: w447 -> [w450 _]
              frame "None", Default {
                # ">> WIill proceed to part ii if not manual override >>"
                # ">>If ENABLE or Trigger is set to true>>"
                n191 = Or(x=w450, y=w451) -> (x .or. y?=w452:bool)
                n192 = case shown="False" w450 {
                  tunnel: [w463 w469] -> w458
                  tunnel: w457 -> [w462 w468]
                  frame False {
                    n193 = for {
                      shift-right: [w465] -> w463
                      shift-left: w462 -> [w466]
                      tunnel: string[] ["Z STEPPER CAM HEIGHT", "READ STEPPER VALUES"] ("element") -> [w464] mode=indexing
                      n194 = Enqueue Element(queue=w466, element=w464) -> (queue out=w465:refnum<queue>)  [unwired: 2 in, 2 out]
                    }
                  }
                  frame True {
                    n195 = for {
                      shift-right: [w471] -> w469
                      shift-left: w468 -> [w472]
                      tunnel: string[] ["ARDUINO - ULTRASONIC", "READ ULTRASONIC", "", "", "", ""] -> [w470] mode=indexing
                      n196 = Enqueue Element(queue=w472, element=w470) -> (queue out=w471:refnum<queue>)  [unwired: 2 in, 2 out]
                    }
                  }
                }
                n197 = Select(t=State_Type_Definitions."True Stop" ("Enum"), s=w451, f=State_Type_Definitions."Task 2:Sensor Mode" ("Enum")) -> (s? t:f=w454:T6)
                n198 = Select(t=w454, s=w452, f=State_Type_Definitions."Task 2:Raise Arm" ("Enum")) -> (s? t:f=w460:T6)
              }
              frame "Exit" {
                n199 = for {
                  shift-right: [w478] -> w475
                  shift-left: _ -> [w479]
                  tunnel: string[] ["STOP", "RESET ENCODERS", "RESET YAW", ""] -> [w477] mode=indexing
                  n200 = Enqueue Element(queue=w479, element=w477) -> (queue out=w478:refnum<queue>)  [unwired: 2 in, 2 out]
                }
              }
            }
          }
          frame 9 {
            w494 = u8 30 ("y")
            # ">>> yStepper command>>>"
            # ">>Object detected>>"
            n201 = Dequeue Element(queue=w486, timeout in ms (-1)=w485, error in (no error)=w484) -> (element=w495:T7)  [unwired: 3 out]
            n202 = Less?(x=w482, y=w494) -> (x < y?=w493:bool)
            n203 = Less?(x=w481, y=w494) -> (x < y?=w492:bool)
            n204 = Or(x=w493, y=w492) -> (x .or. y?=w491:bool)
            "Obstacle detected" <- w491
            n205 = case shown="\"None\", Default" w495 {
              tunnel: w491 -> [w499 _]
              tunnel: [w501 State_Type_Definitions."True Stop" ("Enum")] -> w490
              tunnel: w483 -> [w500 _]
              tunnel: w487 -> [w498 w518]
              tunnel: [w497 w519] -> w489
              tunnel: [State_Type_Definitions."Idle" ("Enum") State_Type_Definitions."Shutdown" ("Enum")] -> w488
              frame "None", Default {
                n206 = case shown="True" w499 {
                  tunnel: w498 -> [w505 w512]
                  tunnel: [w506 w511] -> w497
                  frame False {
                    n207 = for {
                      tunnel: string[] ["READ ULTRASONIC", "STOP"] ("element") -> [w507] mode=indexing
                      shift-right: [w509] -> w506
                      shift-left: w505 -> [w508]
                      n208 = Enqueue Element(queue=w508, element=w507) -> (queue out=w509:refnum<queue>)  [unwired: 2 in, 2 out]
                    }
                  }
                  frame True {
                    n209 = for {
                      shift-right: [w514] -> w511
                      shift-left: w512 -> [w515]
                      tunnel: string[] ["REVERSE", "READ ULTRASONIC", "READ YAW"] -> [w513] mode=indexing
                      n210 = Enqueue Element(queue=w515, element=w513) -> (queue out=w514:refnum<queue>)  [unwired: 2 in, 2 out]
                    }
                  }
                }
                n211 = Select(t=State_Type_Definitions."True Stop" ("Enum"), s=w500, f=State_Type_Definitions."Task 2:Sensor Mode" ("Enum")) -> (s? t:f=w501:T6)
              }
              frame "Exit" {
                n212 = for {
                  shift-right: [w522] -> w519
                  shift-left: w518 -> [w523]
                  tunnel: string[] ["STOP", "RESET ENCODERS", "RESET YAW", "ARDUINO MODE 0"] -> [w521] mode=indexing
                  n213 = Enqueue Element(queue=w523, element=w521) -> (queue out=w522:refnum<queue>)  [unwired: 2 in, 2 out]
                }
              }
            }
          }
          frame 11 {
            # ">>> yStepper command>>>"
            n214 = Dequeue Element(queue=w537, timeout in ms (-1)=w536, error in (no error)=w535) -> (element=w526:T7)  [unwired: 3 out]
            n215 = Greater?(x=w534, y=160.0) -> (0:w531:bool)
            n216 = Or(x=w531, y=w532) -> (x .or. y?=w527:bool)
            n217 = case shown="\"None\", Default" w526 {
              tunnel: w527 -> [w540 _]
              tunnel: [w544 State_Type_Definitions."True Stop" ("Enum")] -> w528
              tunnel: w530 -> [w541 w560]
              tunnel: [w539 w559] -> w529
              tunnel: [State_Type_Definitions."Idle" ("Enum") State_Type_Definitions."Shutdown" ("Enum")] -> w525
              frame "None", Default {
                n218 = case shown="False" w540 {
                  tunnel: w541 -> [w547 w553]
                  tunnel: [w546 w551] -> w539
                  frame False {
                    n219 = for {
                      shift-right: [w549] -> w546
                      shift-left: w547 -> [w550]
                      tunnel: string[] ["READ ENCODERS", "R-ACW"] ("element") -> [w548] mode=indexing
                      n220 = Enqueue Element(queue=w550, element=w548) -> (queue out=w549:refnum<queue>)  [unwired: 2 in, 2 out]
                    }
                  }
                  frame True {
                    n221 = for {
                      shift-right: [w555] -> w551
                      shift-left: w553 -> [w556]
                      tunnel: string[] ["RESET YAW", "RESET ENCODERS", "STOP", "ARDUINO MODE 0"] -> [w554] mode=indexing
                      n222 = Enqueue Element(queue=w556, element=w554) -> (queue out=w555:refnum<queue>)  [unwired: 2 in, 2 out]
                    }
                  }
                }
                n223 = Select(t=State_Type_Definitions."True Stop" ("Enum"), s=w540, f=State_Type_Definitions."Task 3" ("Enum")) -> (s? t:f=w544:T6)
              }
              frame "Exit" {
                n224 = for {
                  shift-right: [w563] -> w559
                  shift-left: w560 -> [w564]
                  tunnel: string[] ["STOP", "RESET ENCODERS", "RESET YAW", ""] -> [w562] mode=indexing
                  n225 = Enqueue Element(queue=w564, element=w562) -> (queue out=w563:refnum<queue>)  [unwired: 2 in, 2 out]
                }
              }
            }
          }
          frame 12 {
            # ">> Stepper height reeached >>"
            # ">>> yStepper command>>>"
            # ">> Manual override >>"
            n226 = Dequeue Element(queue=w576, timeout in ms (-1)=w575, error in (no error)=w574) -> (element=w573:T7)  [unwired: 3 out]
            n227 = Equal?(x=w567, y=u8 80) -> (x = y?=w565:bool)
            n228 = case shown="\"None\", Default" w573 {
              tunnel: [w588 State_Type_Definitions."True Stop" ("Enum")] -> w572
              tunnel: [w586 w603] -> w571
              tunnel: w577 -> [w585 _]
              tunnel: w570 -> [w579 _]
              tunnel: [State_Type_Definitions."Idle" ("Enum") State_Type_Definitions."Shutdown" ("Enum")] -> w569
              tunnel: w565 -> [w578 _]
              frame "None", Default {
                # ">> WIill proceed to part ii if not manual override >>"
                # ">>If ENABLE or Trigger is set to true>>"
                n229 = Or(x=w578, y=w579) -> (x .or. y?=w580:bool)
                n230 = case shown="True" w578 {
                  tunnel: [w591 w597] -> w586
                  tunnel: w585 -> [w590 w596]
                  frame False {
                    n231 = for {
                      shift-right: [w593] -> w591
                      shift-left: w590 -> [w594]
                      tunnel: string[] ["Z STEPPER CAM HEIGHT", "READ STEPPER VALUES"] ("element") -> [w592] mode=indexing
                      n232 = Enqueue Element(queue=w594, element=w592) -> (queue out=w593:refnum<queue>)  [unwired: 2 in, 2 out]
                    }
                  }
                  frame True {
                    n233 = for {
                      shift-right: [w599] -> w597
                      shift-left: w596 -> [w600]
                      tunnel: string[] ["ARDUINO - ULTRASONIC", "READ ULTRASONIC", "FORWARD", "", "", ""] -> [w598] mode=indexing
                      n234 = Enqueue Element(queue=w600, element=w598) -> (queue out=w599:refnum<queue>)  [unwired: 2 in, 2 out]
                    }
                  }
                }
                n235 = Select(t=State_Type_Definitions."True Stop" ("Enum"), s=w579, f=State_Type_Definitions."Task 4_B" ("Enum")) -> (s? t:f=w582:T6)
                n236 = Select(t=w582, s=w580, f=State_Type_Definitions."Task 4_A" ("Enum")) -> (s? t:f=w588:T6)
              }
              frame "Exit" {
                n237 = for {
                  shift-right: [w606] -> w603
                  shift-left: _ -> [w607]
                  tunnel: string[] ["STOP", "RESET ENCODERS", "RESET YAW", ""] -> [w605] mode=indexing
                  n238 = Enqueue Element(queue=w607, element=w605) -> (queue out=w606:refnum<queue>)  [unwired: 2 in, 2 out]
                }
              }
            }
          }
          frame 13 {
            w611 = u8 20
            # ">> Path blocked >>"
            # ">>> yStepper command>>>"
            # ">> Manual override >>"
            n239 = Dequeue Element(queue=w620, timeout in ms (-1)=w619, error in (no error)=w618) -> (element=w617:T7)  [unwired: 3 out]
            n240 = Less?(x=w613, y=w611) -> (x < y?=w608:bool)
            n241 = Less?(x=w612, y=w611) -> (x < y?=w609:bool)
            n242 = And(x=w609, y=w608) -> (x .and. y?=w610:bool)
            n243 = case shown="\"None\", Default" w617 {
              tunnel: [w634 State_Type_Definitions."True Stop" ("Enum")] -> w622
              tunnel: [w632 w649] -> w623
              tunnel: w616 -> [w631 _]
              tunnel: w621 -> [w625 _]
              tunnel: [State_Type_Definitions."Idle" ("Enum") State_Type_Definitions."Shutdown" ("Enum")] -> w615
              tunnel: w610 -> [w624 _]
              frame "None", Default {
                # ">> Manual override forces program to true stop >>"
                # ">>If ENABLE or Trigger is set to true>>"
                n244 = Or(x=w624, y=w625) -> (x .or. y?=w630:bool)
                n245 = case shown="False" w624 {
                  tunnel: [w637 w642] -> w632
                  tunnel: w631 -> [w636 w641]
                  frame False {
                    n246 = for {
                      shift-right: [w639] -> w637
                      shift-left: w636 -> [w640]
                      tunnel: string[] ["FORWARD", "READ ULTRASONIC", "READ YAW"] ("element") -> [w638] mode=indexing
                      n247 = Enqueue Element(queue=w640, element=w638) -> (queue out=w639:refnum<queue>)  [unwired: 2 in, 2 out]
                    }
                  }
                  frame True {
                    n248 = for {
                      shift-right: [w645] -> w642
                      shift-left: w641 -> [w646]
                      tunnel: string[] ["STOP", "RESET YAW", "RESET ENCODERS", "RESET FLAGS"] -> [w644] mode=indexing
                      n249 = Enqueue Element(queue=w646, element=w644) -> (queue out=w645:refnum<queue>)  [unwired: 2 in, 2 out]
                    }
                  }
                }
                n250 = Select(t=State_Type_Definitions."True Stop" ("Enum"), s=w625, f=State_Type_Definitions."Task 4_C" ("Enum")) -> (s? t:f=w627:T6)
                n251 = Select(t=w627, s=w630, f=State_Type_Definitions."Task 4_B" ("Enum")) -> (s? t:f=w634:T6)
              }
              frame "Exit" {
                n252 = for {
                  shift-right: [w652] -> w649
                  shift-left: _ -> [w653]
                  tunnel: string[] ["STOP", "RESET ENCODERS", "RESET YAW", ""] -> [w651] mode=indexing
                  n253 = Enqueue Element(queue=w653, element=w651) -> (queue out=w652:refnum<queue>)  [unwired: 2 in, 2 out]
                }
              }
            }
          }
          frame 14 {
            w663 = u8 20
            # ">> xDistance travelled>>"
            # ">> Path NOT blocked >>"
            # ">>> yStepper command>>>"
            # ">> Manual override >>"
            n254 = Dequeue Element(queue=w673, timeout in ms (-1)=w666, error in (no error)=w665) -> (element=w667:T7)  [unwired: 3 out]
            n255 = Greater?(x=w655, y=w663) -> (0:w661:bool)
            n256 = Greater?(x=w660, y=80.0) -> (0:w658:bool)
            n257 = Greater?(x=w654, y=w663) -> (0:w662:bool)
            n258 = And(x=w662, y=w661) -> (x .and. y?=w657:bool)
            n259 = And(x=w658, y=w657) -> (x .and. y?=w656:bool)
            n260 = case shown="\"None\", Default" w667 {
              tunnel: [w684 State_Type_Definitions."True Stop" ("Enum")] -> w670
              tunnel: [w682 w700] -> w669
              tunnel: w672 -> [w681 w697]
              tunnel: w671 -> [w675 _]
              tunnel: [State_Type_Definitions."Idle" ("t") State_Type_Definitions."Shutdown" ("Enum")] -> w668
              tunnel: w656 -> [w674 _]
              frame "None", Default {
                # ">> Manual override forces program to true stop >>"
                # ">>If ENABLE or Trigger is set to true>>"
                n261 = Or(x=w674, y=w675) -> (x .or. y?=w680:bool)
                n262 = case shown="True" w674 {
                  tunnel: [w687 w692] -> w682
                  tunnel: w681 -> [w685 w691]
                  frame False {
                    n263 = for {
                      shift-right: [w689] -> w687
                      shift-left: w685 -> [w690]
                      tunnel: string[] ["RIGHT", "READ YAW", "READ ENCODERS", "READ ULTRASONIC"] ("element") -> [w688] mode=indexing
                      n264 = Enqueue Element(queue=w690, element=w688) -> (queue out=w689:refnum<queue>)  [unwired: 2 in, 2 out]
                    }
                  }
                  frame True {
                    n265 = for {
                      shift-right: [w695] -> w692
                      shift-left: w691 -> [w696]
                      tunnel: string[] ["STOP", "RESET YAW", "RESET ENCODERS", "ARDUINO - ULTRASONIC"] -> [w694] mode=indexing
                      n266 = Enqueue Element(queue=w696, element=w694) -> (queue out=w695:refnum<queue>)  [unwired: 2 in, 2 out]
                    }
                  }
                }
                n267 = Select(t=State_Type_Definitions."True Stop" ("Enum"), s=w675, f=State_Type_Definitions."Task 4_D" ("Enum")) -> (s? t:f=w676:T6)
                n268 = Select(t=w676, s=w680, f=State_Type_Definitions."Task 4_C" ("Enum")) -> (s? t:f=w684:T6)
              }
              frame "Exit" {
                n269 = for {
                  shift-right: [w703] -> w700
                  shift-left: w697 -> [w704]
                  tunnel: string[] ["STOP", "RESET ENCODERS", "RESET YAW", ""] -> [w702] mode=indexing
                  n270 = Enqueue Element(queue=w704, element=w702) -> (queue out=w703:refnum<queue>)  [unwired: 2 in, 2 out]
                }
              }
            }
          }
          frame 15 {
            w723 = u8 20
            # ">> yDistance travelled>>"
            # ">> Path blocked >>"
            # ">>> yStepper command>>>"
            # ">> Manual override >>"
            n271 = Dequeue Element(queue=w714, timeout in ms (-1)=w713, error in (no error)=w712) -> (element=w724:T7)  [unwired: 3 out]
            n272 = Less?(x=w707, y=w723) -> (x < y?=w721:bool)
            n273 = Greater?(x=w711, y=200.0) -> (0:w719:bool)
            n274 = Less?(x=w706, y=w723) -> (x < y?=w722:bool)
            n275 = And(x=w722, y=w721) -> (x .and. y?=w718:bool)
            n276 = Or(x=w719, y=w718) -> (x .or. y?=w717:bool)
            n277 = case shown="\"None\", Default" w724 {
              tunnel: [w735 State_Type_Definitions."True Stop" ("Enum")] -> w710
              tunnel: [w733 w751] -> w708
              tunnel: w715 -> [w732 w748]
              tunnel: w716 -> [w726 _]
              tunnel: [State_Type_Definitions."Idle" ("t") State_Type_Definitions."Shutdown" ("Enum")] -> w709
              tunnel: w717 -> [w725 _]
              frame "None", Default {
                # ">> Manual override forces program to true stop >>"
                # ">>If ENABLE or Trigger is set to true>>"
                n278 = Or(x=w725, y=w726) -> (x .or. y?=w731:bool)
                n279 = case shown="False" w725 {
                  tunnel: [w738 w743] -> w733
                  tunnel: w732 -> [w736 w742]
                  frame False {
                    n280 = for {
                      shift-right: [w740] -> w738
                      shift-left: w736 -> [w741]
                      tunnel: string[] ["FORWARD", "READ YAW", "READ ENCODERS", "READ ULTRASONIC"] ("element") -> [w739] mode=indexing
                      n281 = Enqueue Element(queue=w741, element=w739) -> (queue out=w740:refnum<queue>)  [unwired: 2 in, 2 out]
                    }
                  }
                  frame True {
                    n282 = for {
                      shift-right: [w746] -> w743
                      shift-left: w742 -> [w747]
                      tunnel: string[] ["STOP", "RESET YAW", "RESET ENCODERS", "RESET FLAGS"] -> [w745] mode=indexing
                      n283 = Enqueue Element(queue=w747, element=w745) -> (queue out=w746:refnum<queue>)  [unwired: 2 in, 2 out]
                    }
                  }
                }
                n284 = Select(t=State_Type_Definitions."True Stop" ("Enum"), s=w726, f=State_Type_Definitions."True Stop" ("Enum")) -> (s? t:f=w727:T6)
                n285 = Select(t=w727, s=w731, f=State_Type_Definitions."Task 4_D" ("Enum")) -> (s? t:f=w735:T6)
              }
              frame "Exit" {
                n286 = for {
                  shift-right: [w754] -> w751
                  shift-left: w748 -> [w755]
                  tunnel: string[] ["STOP", "RESET ENCODERS", "RESET YAW", ""] -> [w753] mode=indexing
                  n287 = Enqueue Element(queue=w755, element=w753) -> (queue out=w754:refnum<queue>)  [unwired: 2 in, 2 out]
                }
              }
            }
          }
          frame 14 {
            # ">>> yStepper command>>>"
            # ">> Manual override >>"
            n288 = Dequeue Element(queue=w764, timeout in ms (-1)=w763, error in (no error)=w765) -> (element=w762:T7)  [unwired: 3 out]
            n289 = Equal?(x=w761, y=u8 80) -> (x = y?=w759:bool)
            n290 = case shown="\"None\", Default" w762 {
              tunnel: [w775 State_Type_Definitions."True Stop" ("Enum")] -> w766
              tunnel: [w778 w795] -> w767
              tunnel: [State_Type_Definitions."Idle" ("Enum") State_Type_Definitions."Shutdown" ("Enum")] -> w768
              tunnel: w759 -> [w774 _]
              tunnel: w758 -> [w773 _]
              tunnel: w757 -> [w769 w792]
              frame "None", Default {
                # "Stays in Task 5_A until stepper reaches desired \nheight"
                # "T: Go back to idle, F: Continue with task\""
                # ">> Manual override >>"
                n291 = case shown="True" w774 {
                  tunnel: [w782 w788] -> w778
                  tunnel: w769 -> [w780 w786]
                  frame False {
                    n292 = for {
                      tunnel: string[] ["Z STEPPER CAM HEIGHT", "READ STEPPER VALUES"] ("element") -> [w783] mode=indexing
                      shift-right: [w785] -> w782
                      shift-left: w780 -> [w784]
                      n293 = Enqueue Element(queue=w784, element=w783) -> (queue out=w785:refnum<queue>)  [unwired: 2 in, 2 out]
                    }
                  }
                  frame True {
                    n294 = for {
                      shift-right: [w790] -> w788
                      shift-left: w786 -> [w791]
                      tunnel: string[] ["ARDUINO - ULTRASONIC", "READ ULTRASONIC", ""] -> [w789] mode=indexing
                      n295 = Enqueue Element(queue=w791, element=w789) -> (queue out=w790:refnum<queue>)  [unwired: 2 in, 2 out]
                    }
                  }
                }
                n296 = Or(x=w774, y=w773) -> (x .or. y?=w776:bool)
                n297 = Select(t=State_Type_Definitions."True Stop" ("Enum"), s=w773, f=State_Type_Definitions."Task 5 _B" ("Enum")) -> (s? t:f=w770:u16)
                n298 = Select(t=w770, s=w776, f=State_Type_Definitions."Task 5_A" ("Enum")) -> (s? t:f=w775:u16)
              }
              frame "Exit" {
                n299 = for {
                  shift-right: [w798] -> w795
                  shift-left: w792 -> [w799]
                  tunnel: string[] ["STOP", "RESET ENCODERS", "RESET YAW", "ARDUINO MODE 0"] -> [w797] mode=indexing
                  n300 = Enqueue Element(queue=w799, element=w797) -> (queue out=w798:refnum<queue>)  [unwired: 2 in, 2 out]
                }
              }
            }
          }
          frame 15 {
            w805 = u8 20 ("y")
            # ">>> yStepper command>>>"
            n301 = Less?(x=w802, y=w805) -> (x < y?=w803:bool)
            n302 = Dequeue Element(queue=w809, timeout in ms (-1)=w808, error in (no error)=w810) -> (element=w807:T7)  [unwired: 3 out]
            n303 = Less?(x=w801, y=w805) -> (x < y?=w804:bool)
            n304 = And(x=w804, y=w803) -> (x .and. y?=w800:bool)
            n305 = case shown="\"None\", Default" w807 {
              tunnel: [w822 State_Type_Definitions."True Stop" ("Enum")] -> w812
              tunnel: [w825 w842] -> w811
              tunnel: [State_Type_Definitions."Idle" ("Enum") State_Type_Definitions."Shutdown" ("Enum")] -> w813
              tunnel: w815 -> [w821 _]
              tunnel: w814 -> [w817 w839]
              tunnel: w800 -> [w816 _]
              frame "None", Default {
                # "Stays in Task 5_B to capture image over 5 seconds"
                # "T: Go back to idle, F: Continue with task\""
                # ">> Manual override >>"
                n306 = case shown="True" w816 {
                  tunnel: [w829 w835] -> w825
                  tunnel: w817 -> [w827 w833]
                  frame False {
                    n307 = for {
                      tunnel: string[] ["FORWARD", "READ ULTRASONIC", "READ YAW"] ("element") -> [w830] mode=indexing
                      shift-right: [w832] -> w829
                      shift-left: w827 -> [w831]
                      n308 = Enqueue Element(queue=w831, element=w830) -> (queue out=w832:refnum<queue>)  [unwired: 2 in, 2 out]
                    }
                  }
                  frame True {
                    n309 = for {
                      shift-right: [w837] -> w835
                      shift-left: w833 -> [w838]
                      tunnel: string[] ["STOP", "RESET ENCODERS", "OPEN LOG CAM", "SET TIMER"] -> [w836] mode=indexing
                      n310 = Enqueue Element(queue=w838, element=w836) -> (queue out=w837:refnum<queue>)  [unwired: 2 in, 2 out]
                    }
                  }
                }
                n311 = Or(x=w816, y=w821) -> (x .or. y?=w823:bool)
                n312 = Select(t=State_Type_Definitions."True Stop" ("Enum"), s=w821, f=State_Type_Definitions."Task 5_C" ("Enum")) -> (s? t:f=w818:u16)
                n313 = Select(t=w818, s=w823, f=State_Type_Definitions."Task 5 _B" ("Enum")) -> (s? t:f=w822:u16)
              }
              frame "Exit" {
                n314 = for {
                  shift-right: [w845] -> w842
                  shift-left: w839 -> [w846]
                  tunnel: string[] ["STOP", "RESET ENCODERS", "RESET YAW", "ARDUINO MODE 0"] -> [w844] mode=indexing
                  n315 = Enqueue Element(queue=w846, element=w844) -> (queue out=w845:refnum<queue>)  [unwired: 2 in, 2 out]
                }
              }
            }
          }
          frame 16 {
            # ">>> yStepper command>>>"
            # ">> Manual override >>"
            n316 = Dequeue Element(queue=w855, timeout in ms (-1)=w854, error in (no error)=w853) -> (element=w852:T7)  [unwired: 3 out]
            n317 = case shown="\"None\", Default" w852 {
              tunnel: [w862 State_Type_Definitions."True Stop" ("Enum")] -> w857
              tunnel: [w865 w882] -> w850
              tunnel: [State_Type_Definitions."Idle" ("Enum") State_Type_Definitions."Shutdown" ("Enum")] -> w849
              tunnel: w851 -> [w859 _]
              tunnel: w856 -> [w861 w879]
              tunnel: w847 -> [w858 _]
              frame "None", Default {
                # ">> Is time up? >>"
                # "Determines if object is in range to pick up"
                # ">> Manual override >>"
                n318 = case shown="True" w858 {
                  tunnel: [w869 w875] -> w865
                  tunnel: w861 -> [w867 w873]
                  frame False {
                    n319 = for {
                      tunnel: string[] ["CAM ACQ", "START TIMER"] ("element") -> [w870] mode=indexing
                      shift-right: [w872] -> w869
                      shift-left: w867 -> [w871]
                      n320 = Enqueue Element(queue=w871, element=w870) -> (queue out=w872:refnum<queue>)  [unwired: 2 in, 2 out]
                    }
                  }
                  frame True {
                    n321 = for {
                      shift-right: [w877] -> w875
                      shift-left: w873 -> [w878]
                      tunnel: string[] ["CAM CLOSE", "PROCESS IMAGE"] -> [w876] mode=indexing
                      n322 = Enqueue Element(queue=w878, element=w876) -> (queue out=w877:refnum<queue>)  [unwired: 2 in, 2 out]
                    }
                  }
                }
                n323 = Or(x=w858, y=w859) -> (x .or. y?=w863:bool)
                n324 = Select(t=State_Type_Definitions."Task 5_D" ("Enum"), s=w863, f=State_Type_Definitions."Task 5_D" ("Enum")) -> (s? t:f=w862:T24)
              }
              frame "Exit" {
                n325 = for {
                  shift-right: [w885] -> w882
                  shift-left: w879 -> [w886]
                  tunnel: string[] ["STOP", "RESET ENCODERS", "RESET YAW", "ARDUINO MODE 0"] -> [w884] mode=indexing
                  n326 = Enqueue Element(queue=w886, element=w884) -> (queue out=w885:refnum<queue>)  [unwired: 2 in, 2 out]
                }
              }
            }
          }
          frame 17 {
            # ">>> yStepper command>>>"
            n327 = Dequeue Element(queue=w892, timeout in ms (-1)=w891, error in (no error)=w890) -> (element=w889:T7)  [unwired: 3 out]
            n328 = case shown="\"None\", Default" w889 {
              tunnel: [w904 State_Type_Definitions."True Stop" ("Enum")] -> w896
              tunnel: [w907 w924] -> w895
              tunnel: [State_Type_Definitions."Idle" ("Enum") State_Type_Definitions."Shutdown" ("Enum")] -> w897
              tunnel: w893 -> [w903 _]
              tunnel: w894 -> [w899 w921]
              tunnel: w887 -> [w898 _]
              frame "None", Default {
                # ">> T: Breaks out of state loop; F: Stays in loop>>"
                # ">> Manual override >>"
                # ">> Checks if object is detected>>"
                # "Stays in Task 5D until the object is detected"
                # "T: Go back to idle, F: Continue with task\""
                # ">> Manual override >>"
                n329 = case shown="False" w898 {
                  tunnel: [w911 w917] -> w907
                  tunnel: w899 -> [w909 w915]
                  frame False {
                    n330 = for {
                      tunnel: string[] ["PROCESS IMAGE", "", ""] ("element") -> [w912] mode=indexing
                      shift-right: [w914] -> w911
                      shift-left: w909 -> [w913]
                      n331 = Enqueue Element(queue=w913, element=w912) -> (queue out=w914:refnum<queue>)  [unwired: 2 in, 2 out]
                    }
                  }
                  frame True {
                    n332 = for {
                      shift-right: [w919] -> w917
                      shift-left: w915 -> [w920]
                      tunnel: string[] ["DISPOSE BUFFERS", "CAM CLOSE", ""] -> [w918] mode=indexing
                      n333 = Enqueue Element(queue=w920, element=w918) -> (queue out=w919:refnum<queue>)  [unwired: 2 in, 2 out]
                    }
                  }
                }
                n334 = Or(x=w898, y=w903) -> (x .or. y?=w905:bool)
                n335 = Select(t=State_Type_Definitions."True Stop" ("Enum"), s=w903, f=State_Type_Definitions."True Stop" ("Enum")) -> (s? t:f=w900:T6)
                n336 = Select(t=w900, s=w905, f=State_Type_Definitions."Task 5_D" ("Enum")) -> (s? t:f=w904:u16)
              }
              frame "Exit" {
                n337 = for {
                  shift-right: [w927] -> w924
                  shift-left: w921 -> [w928]
                  tunnel: string[] ["STOP", "RESET ENCODERS", "RESET YAW", "ARDUINO MODE 0"] -> [w926] mode=indexing
                  n338 = Enqueue Element(queue=w928, element=w926) -> (queue out=w927:refnum<queue>)  [unwired: 2 in, 2 out]
                }
              }
            }
          }
          frame 24 {
            # ">>> yStepper command>>>"
            n339 = Dequeue Element(queue=w936, timeout in ms (-1)=w935, error in (no error)=w934) -> (element=w941:T7)  [unwired: 3 out]
            n340 = Equal?(x=w932, y=u8 80) -> (x = y?=w931:bool)
            n341 = case shown="\"None\", Default" w941 {
              tunnel: [w948 State_Type_Definitions."True Stop" ("Enum")] -> w939
              tunnel: [w947 w965] -> w938
              tunnel: [State_Type_Definitions."Idle" ("Enum") State_Type_Definitions."Shutdown" ("Enum")] -> w940
              tunnel: w937 -> [w943 _]
              tunnel: w933 -> [w945 _]
              tunnel: w931 -> [w942 _]
              frame "None", Default {
                n342 = case shown="False" w942 {
                  tunnel: [w953 w959] -> w947
                  tunnel: w945 -> [w951 w957]
                  frame False {
                    n343 = for {
                      tunnel: string[] ["Z STEPPER CAM HEIGHT", "READ STEPPER VALUES"] ("element") -> [w954] mode=indexing
                      shift-right: [w956] -> w953
                      shift-left: w951 -> [w955]
                      n344 = Enqueue Element(queue=w955, element=w954) -> (queue out=w956:refnum<queue>)  [unwired: 2 in, 2 out]
                    }
                  }
                  frame True {
                    n345 = for {
                      shift-right: [w961] -> w959
                      shift-left: w957 -> [w962]
                      tunnel: string[] ["CAM ACQ", "OPEN LOG CAM"] -> [w960] mode=indexing
                      n346 = Enqueue Element(queue=w962, element=w960) -> (queue out=w961:refnum<queue>)  [unwired: 2 in, 2 out]
                    }
                  }
                }
                n347 = Or(x=w942, y=w943) -> (x .or. y?=w944:bool)
                n348 = Select(t=State_Type_Definitions."Task 6_B" ("Enum"), s=w944, f=State_Type_Definitions."Task 6_A" ("Enum")) -> (s? t:f=w948:T6)
              }
              frame "Exit" {
                n349 = for {
                  shift-right: [w968] -> w965
                  shift-left: _ -> [w969]
                  tunnel: string[] ["STOP", "RESET ENCODERS", "RESET YAW", "ARDUINO MODE 0"] -> [w967] mode=indexing
                  n350 = Enqueue Element(queue=w969, element=w967) -> (queue out=w968:refnum<queue>)  [unwired: 2 in, 2 out]
                }
              }
            }
          }
          frame 25 {
            # ">>> yStepper command>>>"
            n351 = Dequeue Element(queue=w979, timeout in ms (-1)=w977, error in (no error)=w978) -> (element=w976:T7)  [unwired: 3 out]
            n352 = case shown="\"None\", Default" w976 {
              tunnel: [w986 State_Type_Definitions."True Stop" ("Enum")] -> w972
              tunnel: [w985 w1004] -> w980
              tunnel: [State_Type_Definitions."Idle" ("Enum") State_Type_Definitions."Shutdown" ("Enum")] -> w973
              tunnel: w975 -> [w981 _]
              tunnel: w974 -> [w983 _]
              tunnel: w971 -> [w982 w1001]
              frame "None", Default {
                # ">> Manual override >>"
                n353 = case shown="True" w983 {
                  tunnel: [w991 w997] -> w985
                  tunnel: w982 -> [w990 w995]
                  frame False {
                    n354 = for {
                      shift-right: [w994] -> w991
                      shift-left: w990 -> [w993]
                      tunnel: string[] ["CAM ACQ", "PROCESS IMAGE", "OPEN CLAW"] -> [w992] mode=indexing
                      n355 = Enqueue Element(queue=w993, element=w992) -> (queue out=w994:refnum<queue>)  [unwired: 2 in, 2 out]
                    }
                  }
                  frame True {
                    n356 = for {
                      shift-right: [w999] -> w997
                      shift-left: w995 -> [w1000]
                      tunnel: string[] ["CAM ACQ", "PROCESS IMAGE", "CLOSE CLAW"] -> [w998] mode=indexing
                      n357 = Enqueue Element(queue=w1000, element=w998) -> (queue out=w999:refnum<queue>)  [unwired: 2 in, 2 out]
                    }
                  }
                }
                n358 = Select(t=State_Type_Definitions."True Stop" ("Enum"), s=w981, f=State_Type_Definitions."Task 6_B" ("Enum")) -> (s? t:f=w986:T6)
              }
              frame "Exit" {
                # ">> State after true stop >>"
                # ">> Goes to true stop >>"
                n359 = for {
                  shift-right: [w1007] -> w1004
                  shift-left: w1001 -> [w1008]
                  tunnel: string[] ["STOP", "RESET ENCODERS", "RESET YAW", ""] -> [w1006] mode=indexing
                  n360 = Enqueue Element(queue=w1008, element=w1006) -> (queue out=w1007:refnum<queue>)  [unwired: 2 in, 2 out]
                }
              }
            }
          }
          frame 38 {
            # ">> Stepper height reeached >>"
            # ">>> yStepper command>>>"
            # ">> Manual override >>"
            n361 = Dequeue Element(queue=w1018, timeout in ms (-1)=w1013, error in (no error)=w1017) -> (element=w1021:T7)  [unwired: 3 out]
            n362 = Equal?(x=w1015, y=u8 80) -> (x = y?=w1019:bool)
            n363 = case shown="\"None\", Default" w1021 {
              tunnel: [w1032 State_Type_Definitions."True Stop" ("Enum")] -> w1011
              tunnel: [w1030 w1047] -> w1010
              tunnel: w1014 -> [w1029 _]
              tunnel: w1016 -> [w1023 _]
              tunnel: [State_Type_Definitions."Idle" ("Enum") State_Type_Definitions."Shutdown" ("Enum")] -> w1012
              tunnel: w1019 -> [w1022 _]
              frame "None", Default {
                # ">> WIill proceed to part ii if not manual override >>"
                # ">>If ENABLE or Trigger is set to true>>"
                n364 = Or(x=w1022, y=w1023) -> (x .or. y?=w1024:bool)
                n365 = case shown="True" w1022 {
                  tunnel: [w1035 w1041] -> w1030
                  tunnel: w1029 -> [w1034 w1040]
                  frame False {
                    n366 = for {
                      shift-right: [w1037] -> w1035
                      shift-left: w1034 -> [w1038]
                      tunnel: string[] ["Z STEPPER CAM HEIGHT", "READ STEPPER VALUES"] ("element") -> [w1036] mode=indexing
                      n367 = Enqueue Element(queue=w1038, element=w1036) -> (queue out=w1037:refnum<queue>)  [unwired: 2 in, 2 out]
                    }
                  }
                  frame True {
                    n368 = for {
                      shift-right: [w1043] -> w1041
                      shift-left: w1040 -> [w1044]
                      tunnel: string[] ["ARDUINO - ULTRASONIC", "READ ULTRASONIC", "", "", "", ""] -> [w1042] mode=indexing
                      n369 = Enqueue Element(queue=w1044, element=w1042) -> (queue out=w1043:refnum<queue>)  [unwired: 2 in, 2 out]
                    }
                  }
                }
                n370 = Select(t=State_Type_Definitions."True Stop" ("Enum"), s=w1023, f=State_Type_Definitions."Task 9B: Rotate to Angle" ("Enum")) -> (s? t:f=w1026:T6)
                n371 = Select(t=w1026, s=w1024, f=State_Type_Definitions."Task 9A: Raise Arm" ("Enum")) -> (s? t:f=w1032:T6)
              }
              frame "Exit" {
                n372 = for {
                  shift-right: [w1050] -> w1047
                  shift-left: _ -> [w1051]
                  tunnel: string[] ["STOP", "RESET ENCODERS", "RESET YAW", ""] -> [w1049] mode=indexing
                  n373 = Enqueue Element(queue=w1051, element=w1049) -> (queue out=w1050:refnum<queue>)  [unwired: 2 in, 2 out]
                }
              }
            }
          }
          frame 39 {
            # ">>> yStepper command>>>"
            n374 = Dequeue Element(queue=w1063, timeout in ms (-1)=w1062, error in (no error)=w1061) -> (element=w1065:T7)  [unwired: 3 out]
            n375 = In Range and Coerce(upper limit=310.0, x=w1055, lower limit=300.0) -> (In Range?=w1052:bool)  [unwired: 1 out]
            n376 = case shown="\"None\", Default" w1065 {
              tunnel: w1056 -> [w1068 _]
              tunnel: [w1076 State_Type_Definitions."True Stop" ("Enum")] -> w1058
              tunnel: w1064 -> [w1074 w1092]
              tunnel: [w1073 w1091] -> w1057
              tunnel: [State_Type_Definitions."Idle" ("Enum") State_Type_Definitions."Shutdown" ("Enum")] -> w1059
              tunnel: w1052 -> [w1066 _]
              frame "None", Default {
                n377 = Or(x=w1066, y=w1068) -> (x .or. y?=w1067:bool)
                n378 = case shown="True" w1066 {
                  tunnel: w1074 -> [w1079 w1085]
                  tunnel: [w1078 w1083] -> w1073
                  frame False {
                    n379 = for {
                      shift-right: [w1081] -> w1078
                      shift-left: w1079 -> [w1082]
                      tunnel: string[] ["READ YAW", "R-ACW"] ("element") -> [w1080] mode=indexing
                      n380 = Enqueue Element(queue=w1082, element=w1080) -> (queue out=w1081:refnum<queue>)  [unwired: 2 in, 2 out]
                    }
                  }
                  frame True {
                    n381 = for {
                      shift-right: [w1087] -> w1083
                      shift-left: w1085 -> [w1088]
                      tunnel: string[] ["STOP", "RESET ENCODERS", "RESET YAW", ""] -> [w1086] mode=indexing
                      n382 = Enqueue Element(queue=w1088, element=w1086) -> (queue out=w1087:refnum<queue>)  [unwired: 2 in, 2 out]
                    }
                  }
                }
                n383 = Select(t=State_Type_Definitions."True Stop" ("Enum"), s=w1068, f=State_Type_Definitions."Task 9C: Rotation alignmnet") -> (s? t:f=w1070:u16)
                n384 = Select(t=w1070, s=w1067, f=State_Type_Definitions."Task 9B: Rotate to Angle" ("Enum")) -> (s? t:f=w1076:u16)
              }
              frame "Exit" {
                n385 = for {
                  shift-right: [w1095] -> w1091
                  shift-left: w1092 -> [w1096]
                  tunnel: string[] ["STOP", "RESET ENCODERS", "RESET YAW", ""] -> [w1094] mode=indexing
                  n386 = Enqueue Element(queue=w1096, element=w1094) -> (queue out=w1095:refnum<queue>)  [unwired: 2 in, 2 out]
                }
              }
            }
          }
          frame 33 {
            # ">>> yStepper command>>>"
            n387 = Dequeue Element(queue=w1105, timeout in ms (-1)=w1104, error in (no error)=w1103) -> (element=w1106:T7)  [unwired: 3 out]
            n388 = case shown="\"None\", Default" w1106 {
              tunnel: w1101 -> [w1107 _]
              tunnel: [w1115 State_Type_Definitions."True Stop" ("Enum")] -> w1098
              tunnel: w1102 -> [w1113 w1131]
              tunnel: [w1112 w1130] -> w1097
              tunnel: [State_Type_Definitions."Idle" ("Enum") State_Type_Definitions."Shutdown" ("Enum")] -> w1100
              frame "None", Default {
                n389 = case shown="True" w1107 {
                  tunnel: w1113 -> [w1118 w1124]
                  tunnel: [w1117 w1122] -> w1112
                  frame False {
                    n390 = for {
                      shift-right: [w1120] -> w1117
                      shift-left: w1118 -> [w1121]
                      tunnel: string[] ["READ IR", "FORWARD - IR ASSIST"] ("element") -> [w1119] mode=indexing
                      n391 = Enqueue Element(queue=w1121, element=w1119) -> (queue out=w1120:refnum<queue>)  [unwired: 2 in, 2 out]
                    }
                  }
                  frame True {
                    n392 = for {
                      shift-right: [w1126] -> w1122
                      shift-left: w1124 -> [w1127]
                      tunnel: string[] ["STOP", "RESET ENCODERS", "RESET YAW", ""] -> [w1125] mode=indexing
                      n393 = Enqueue Element(queue=w1127, element=w1125) -> (queue out=w1126:refnum<queue>)  [unwired: 2 in, 2 out]
                    }
                  }
                }
                n394 = Select(t=State_Type_Definitions."True Stop" ("Enum"), s=w1107, f=State_Type_Definitions."True Stop") -> (s? t:f=w1109:T6)
                n395 = Select(t=w1109, s=w1107, f=State_Type_Definitions."Task 9C: Rotation alignmnet" ("Enum")) -> (s? t:f=w1115:u16)
              }
              frame "Exit" {
                n396 = for {
                  shift-right: [w1134] -> w1130
                  shift-left: w1131 -> [w1135]
                  tunnel: string[] ["STOP", "RESET ENCODERS", "RESET YAW", ""] -> [w1133] mode=indexing
                  n397 = Enqueue Element(queue=w1135, element=w1133) -> (queue out=w1134:refnum<queue>)  [unwired: 2 in, 2 out]
                }
              }
            }
          }
        }
      }
    }
    n398 = local write "Green LED"(w199) -> ()
  }
  n399 = call <vilib>:"DIO Close.vi"("error in (no error)"=w25, "DIO Info In"=w28) -> ()  [unwired: 9 in, 1 out]
  n400 = call <vilib>:"DIO Close.vi"("error in (no error)"=w35, "DIO Info In"=w37) -> ()  [unwired: 9 in, 1 out]
  n401 = call <vilib>:"NavX Close.vi"("error in (no error)"=w6, "NavX Info In"=w5) -> ()  [unwired: 9 in, 1 out]
  n402 = call <vilib>:"DIO Close.vi"("error in (no error)"=w30, "DIO Info In"=w32) -> ()  [unwired: 9 in, 1 out]
  n403 = call <vilib>:"DIO Close.vi"("error in (no error)"=w13, "DIO Info In"=w14) -> ()  [unwired: 9 in, 1 out]
  n404 = call <vilib>:"DIO Close.vi"("error in (no error)"=w8, "DIO Info In"=w9) -> ()  [unwired: 9 in, 1 out]
  n405 = while {
    stop <- w1635 stop-if-true
    n406 = call <vilib>:"RT Get CPU Loads.vi"() -> ("CPU loads"=→"CPU loads":T5[])  [unwired: 10 in, 1 out]
    n407 = Wait (ms)(milliseconds to wait=u32 100) -> ()  [unwired: 1 out]
    n408 = call "FGV Bool.vi"("Init/Read/Write State"=States_for_Action_Engine."Read") -> ("Output node"=w1635:bool)  [unwired: 2 in, 1 out]
  }
  n409 = while {
    stop <- w1639 stop-if-true
    n410 = call "MOTOR CONTROL WITH PID AE.vi"("AE Mode"=MOTOR_CONTROL_WITH_PID_AE_DATA_MODE_TYPE_DEF."Read from AE") -> ("Speed & distance"=→"Speed & distance":T1)  [unwired: 3 in]
    n411 = call "FGV Bool.vi"("Init/Read/Write State"=States_for_Action_Engine."Read") -> ("Output node"=w1639:bool)  [unwired: 2 in, 1 out]
    n412 = Wait (ms)(milliseconds to wait=u32 5) -> ()  [unwired: 1 out]
  }
  n413 = Merge Errors "Merge Errors"(w65, w64) -> (w47:errorcluster)
  n414 = Merge Errors(w51, w47) -> (w46:errorcluster)
  n415 = Destroy User Event(user event=w68, error in=w46) -> ()  [unwired: 1 out]
  n416 = Destroy User Event(user event=w69, error in=w46) -> ()  [unwired: 1 out]
  n417 = Unregister For Events(event registration refnum=w60, error in=w46) -> ()  [unwired: 1 out]
  n418 = Release Queue(queue=w42, error in (no error)=w46) -> (error out=w24:errorcluster)  [unwired: 1 in, 2 out]
  n419 = Release Queue(queue=w59, error in (no error)=w46) -> ()  [unwired: 1 in, 3 out]
  n420 = call <vilib>:"Simple Error Handler.vi"("error in (no error)"=w24) -> ("error out"=w23:errorcluster)  [unwired: 4 in, 4 out]
  n421 = call <vilib>:"Reset myRIO.vi"("error in (no error)"=w23) -> ("error out"=→"error out":errorcluster)  [unwired: 10 in]
